vi "log table searching.vi"() -> ()   [LabVIEW 2019, in "database.lvlib"]
uses:
  database.lvlib
panel:
  out "Name":string="Search in Database"
  in  "add 5":bool=TRUE
  in  "add 4":bool=TRUE
  in  "add 3":bool=TRUE
  in  "add 2":bool=TRUE
  in  "add 1":bool=TRUE
  in  "sub 5":bool=TRUE
  in  "sub 4":bool=TRUE
  in  "sub 3":bool=TRUE
  in  "sub 2":bool=TRUE
  in  "sub 1":bool=TRUE
  out "Value String 12":string="Value"
  out "Value String 11":string="Value"
  out "Value String 10":string="Value"
  out "Value String 9":string="Value"
  out "Value String 8":string="Value"
  out "Value String 7":string="Value"
  out "Value String 6":string="Value"
  out "Value String 5":string="Value"
  out "Value String 4":string="Value"
  out "Value String 3":string="Value"
  out "Value String 2":string="Value"
  out "Value String 1":string="Value"
  out "String 4":string="Parameter"
  out "String 3":string="Operation"
  out "String 2":string="Value 2"
  out "String 1":string="Value 1"
  in  "Parameter 1":u16(ring) items=["Choose parameter", "Date", "Time", "Catalog ID"]
  in  "Catalog ID 2":u16
  in  "Catalog ID 1":u64
  in  "Time 1":timestamp format="%<%H:%M:%S>T"
  in  "Time 2":timestamp format="%<%H:%M:%S>T"
  in  "Date 1":timestamp format="%<%Y/%m/%d>T"
  in  "Date 2":timestamp format="%<%Y/%m/%d>T"
  in  "Operator 1":u16(ring) items=["All", "P=V1", "P#V1", "P<V1", "P<=V1", "P>V1", "P>=V1", "V1<P<V2", "V1<=P<V2", "V1<P<=V2", "V1<=P<=V2"]
  in  "Parameter 3":u16(ring) items=["Choose parameter", "Date", "Time", "Catalog ID"]
  in  "Parameter 5":u16(ring) items=["Choose parameter", "Date", "Time", "Catalog ID"]
  in  "Parameter 7":u16(ring) items=["Choose parameter", "Date", "Time", "Catalog ID"]
  in  "Parameter 9":u16(ring) items=["Choose parameter", "Date", "Time", "Catalog ID"]
  in  "Parameter 11":u16(ring) items=["Choose parameter", "Date", "Time", "Catalog ID"]
  in  "Operator 3":u16(ring) items=["All", "P=V1", "P#V1", "P<V1", "P<=V1", "P>V1", "P>=V1", "V1<P<V2", "V1<=P<V2", "V1<P<=V2", "V1<=P<=V2"]
  in  "Catalog ID 3":u64
  in  "Catalog ID 4":u16
  in  "Time 3":timestamp format="%<%H:%M:%S>T"
  in  "Time 4":timestamp format="%<%H:%M:%S>T"
  in  "Date 3":timestamp format="%<%Y/%m/%d>T"
  in  "Date 4":timestamp format="%<%Y/%m/%d>T"
  in  "Catalog ID 5":u64
  in  "Catalog ID 6":u16
  in  "Time 5":timestamp format="%<%H:%M:%S>T"
  in  "Time 6":timestamp format="%<%H:%M:%S>T"
  in  "Date 5":timestamp format="%<%Y/%m/%d>T"
  in  "Date 6":timestamp format="%<%Y/%m/%d>T"
  in  "Operator 5":u16(ring) items=["All", "P=V1", "P#V1", "P<V1", "P<=V1", "P>V1", "P>=V1", "V1<P<V2", "V1<=P<V2", "V1<P<=V2", "V1<=P<=V2"]
  in  "Operator 7":u16(ring) items=["All", "P=V1", "P#V1", "P<V1", "P<=V1", "P>V1", "P>=V1", "V1<P<V2", "V1<=P<V2", "V1<P<=V2", "V1<=P<=V2"]
  in  "Catalog ID 7":u64
  in  "Catalog ID 8":u16
  in  "Time 7":timestamp format="%<%H:%M:%S>T"
  in  "Time 8":timestamp format="%<%H:%M:%S>T"
  in  "Date 7":timestamp format="%<%Y/%m/%d>T"
  in  "Date 8":timestamp format="%<%Y/%m/%d>T"
  in  "Catalog ID 9":u64
  in  "Catalog ID 10":u16
  in  "Time 9":timestamp format="%<%H:%M:%S>T"
  in  "Time 10":timestamp format="%<%H:%M:%S>T"
  in  "Date 9":timestamp format="%<%Y/%m/%d>T"
  in  "Date 10":timestamp format="%<%Y/%m/%d>T"
  in  "Catalog ID 11":u64
  in  "Catalog ID 12":u16
  in  "Time 11":timestamp format="%<%H:%M:%S>T"
  in  "Time 12":timestamp format="%<%H:%M:%S>T"
  in  "Date 11":timestamp format="%<%Y/%m/%d>T"
  in  "Date 12":timestamp format="%<%Y/%m/%d>T"
  in  "Operator 11":u16(ring) items=["All", "P=V1", "P#V1", "P<V1", "P<=V1", "P>V1", "P>=V1", "V1<P<V2", "V1<=P<V2", "V1<P<=V2", "V1<=P<=V2"]
  in  "Operator 9":u16(ring) items=["All", "P=V1", "P#V1", "P<V1", "P<=V1", "P>V1", "P>=V1", "V1<P<V2", "V1<=P<V2", "V1<P<=V2", "V1<=P<=V2"]
  in  "Operator 13":u16(ring) items=["AND", "OR"]
  in  "Operator 14":u16(ring) items=["AND", "OR"]
  in  "Operator 15":u16(ring) items=["AND", "OR"]
  in  "Operator 16":u16(ring) items=["AND", "OR"]
  in  "Operator 17":u16(ring) items=["AND", "OR"]
  out "Query String":string
  in  "OK":bool
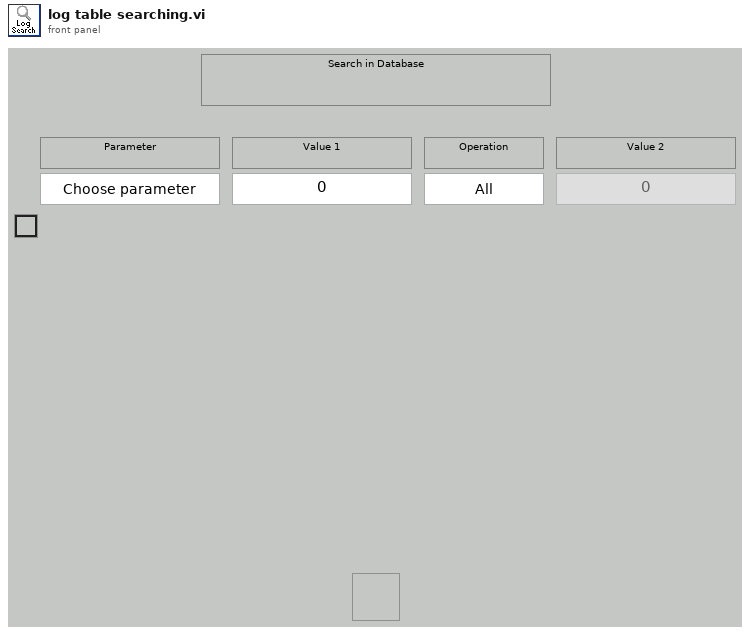
[diagram p1: front panel]
types:
  T1 = enum8{"Enabled", "Disabled", "Disabled and Grayed Out"}
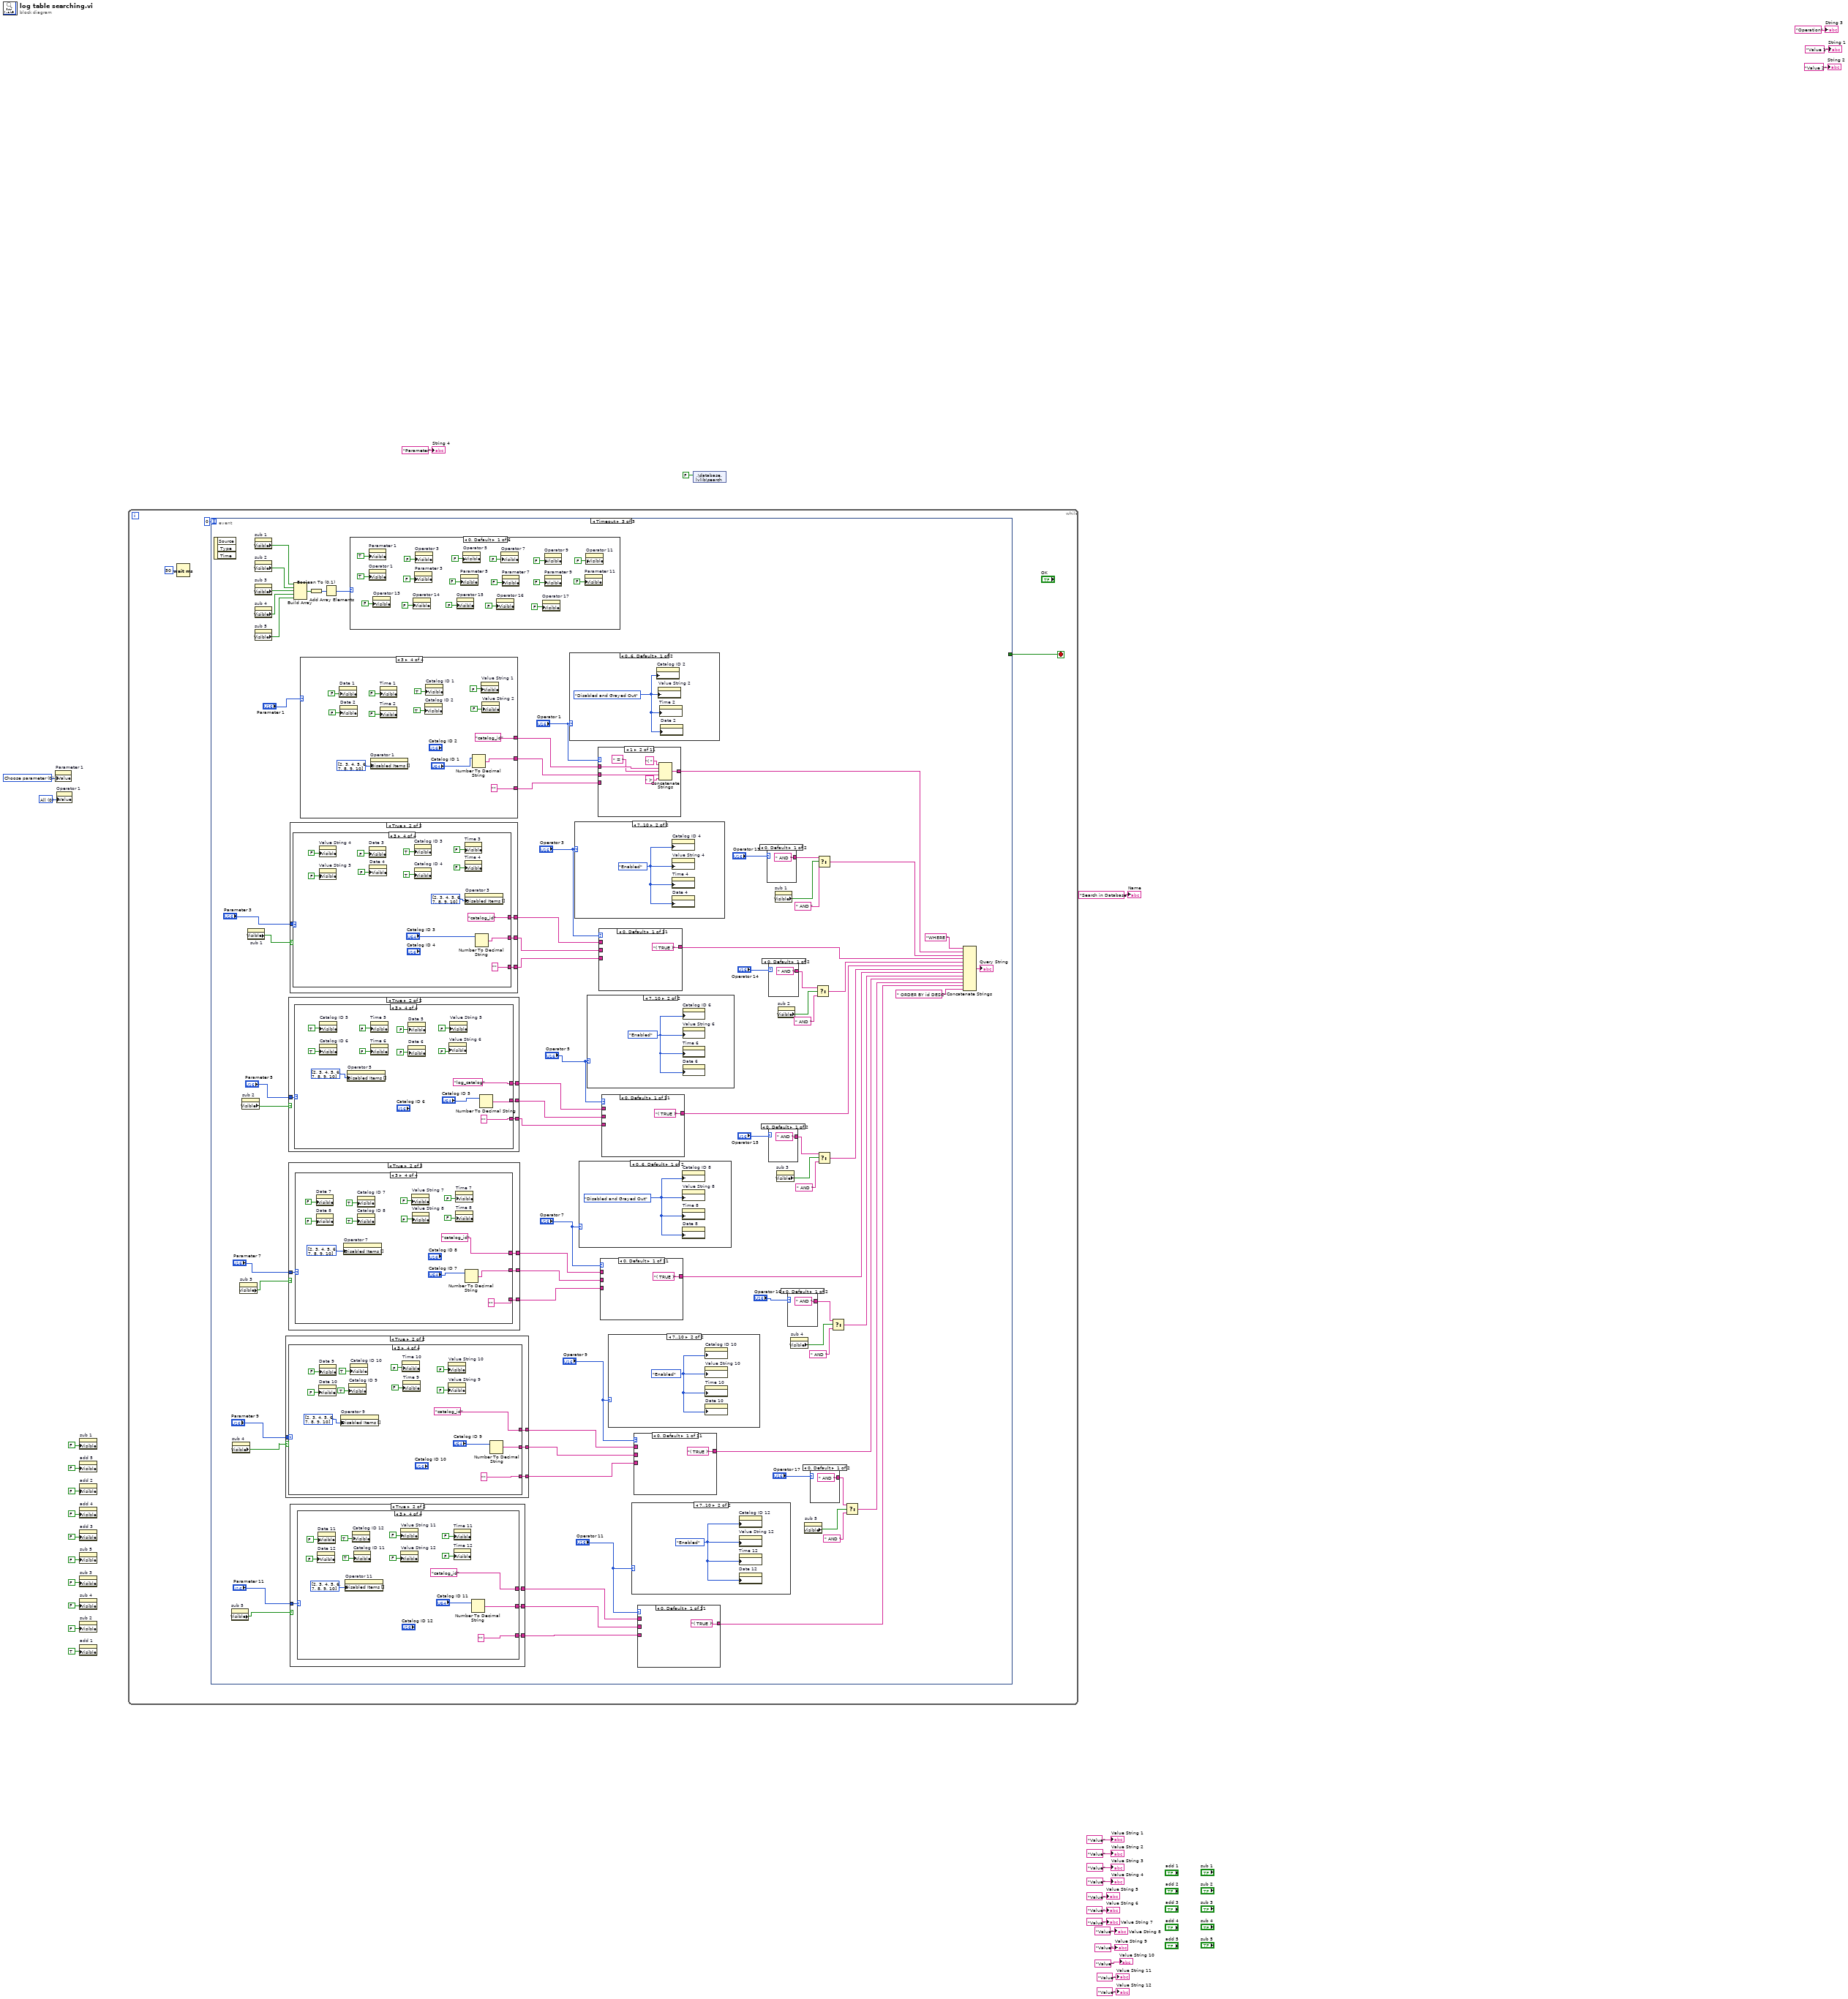
[diagram p0: block diagram]
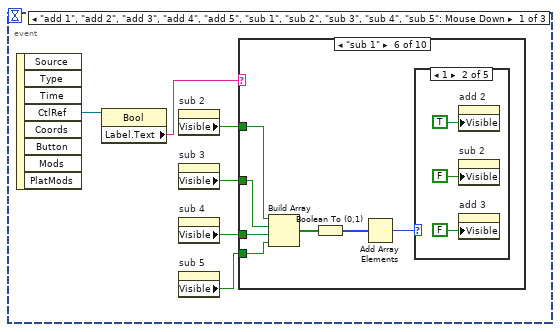
[diagram p2: hidden frame]
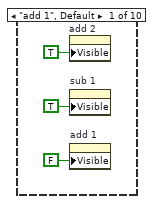
[diagram p3: hidden frame]
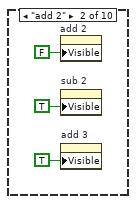
[diagram p4: hidden frame]
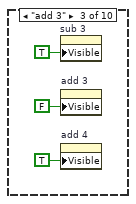
[diagram p5: hidden frame]
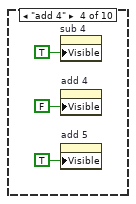
[diagram p6: hidden frame]
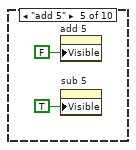
[diagram p7: hidden frame]
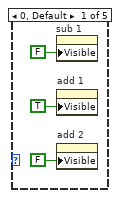
[diagram p8: hidden frame]
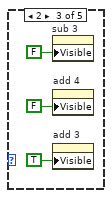
[diagram p9: hidden frame]
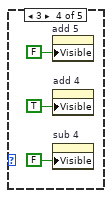
[diagram p10: hidden frame]
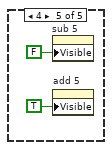
[diagram p11: hidden frame]
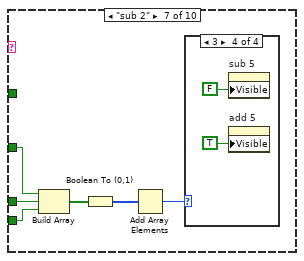
[diagram p12: hidden frame]
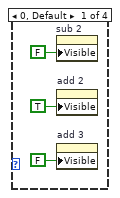
[diagram p13: hidden frame]
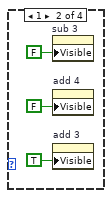
[diagram p14: hidden frame]
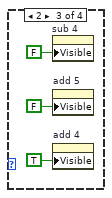
[diagram p15: hidden frame]
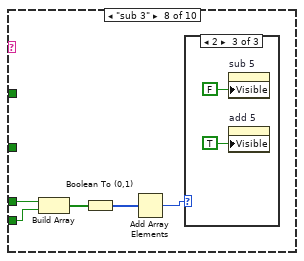
[diagram p16: hidden frame]
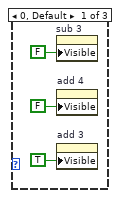
[diagram p17: hidden frame]
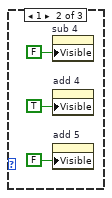
[diagram p18: hidden frame]
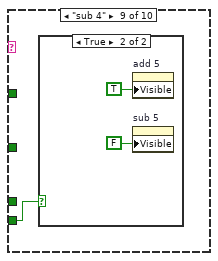
[diagram p19: hidden frame]
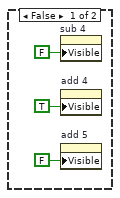
[diagram p20: hidden frame]
diagram:
  w3 = u16 0 items=["All", "P=V1", "P#V1", "P<V1", "P<=V1", "P>V1", "P>=V1", "V1<P<V2", "V1<=P<V2", "V1<P<=V2", "V1<=P<=V2"] ("Operator 1")
  w4 = u16 0 items=["Choose parameter", "Date", "Time", "Disc Situation", "Control Mode", "Camera Situation", "Projector Situation"] ("Parameter 1")
  n1 = property on="Parameter 1" class="Ring (strict)"("Value"=w4) -> ()  [unwired: 2 in, 2 out]
  n2 = property on="Operator 1" class="Ring (strict)"("Value"=w3) -> ()  [unwired: 2 in, 2 out]
  n3 = property on="sub 1" class="Bool"("Visible"=FALSE) -> ()  [unwired: 2 in, 2 out]
  n4 = property on="add 5" class="Bool"("Visible"=FALSE) -> ()  [unwired: 2 in, 2 out]
  n5 = property on="add 2" class="Bool"("Visible"=FALSE) -> ()  [unwired: 2 in, 2 out]
  n6 = property on="add 4" class="Bool"("Visible"=FALSE) -> ()  [unwired: 2 in, 2 out]
  n7 = property on="add 3" class="Bool"("Visible"=FALSE) -> ()  [unwired: 2 in, 2 out]
  n8 = property on="sub 5" class="Bool"("Visible"=FALSE) -> ()  [unwired: 2 in, 2 out]
  n9 = property on="sub 3" class="Bool"("Visible"=FALSE) -> ()  [unwired: 2 in, 2 out]
  n10 = property on="sub 4" class="Bool"("Visible"=FALSE) -> ()  [unwired: 2 in, 2 out]
  n11 = property on="sub 2" class="Bool"("Visible"=FALSE) -> ()  [unwired: 2 in, 2 out]
  n12 = property on="add 1" class="Bool"("Visible"=TRUE) -> ()  [unwired: 2 in, 2 out]
  n13 = while {
    stop <- w31 stop-if-true
    n14 = Wait (ms)(milliseconds to wait=u32 50) -> ()  [unwired: 1 out]
    n15 = event shown="[2] Timeout" {
      selector: _ -> [_ _ _]
      dyn-events: _ -> [_ _ _]
      timeout: 0 -> [_ _ _]
      tunnel: [_ TRUE _] -> w31
      event "add 1", "add 2", "add 3", "add 4", "add 5", "sub 1", "sub 2", "sub 3", "sub 4", "sub 5": Mouse Down {
        n16 = event-data() -> ("CtlRef"=w39:refnum<vi>)  [unwired: 1 in, 7 out]
        n17 = property class="Bool"(reference=w39) -> ("Label.Text"=w38:string)  [unwired: 1 in, 2 out]
        n18 = property on="sub 2" class="Bool"() -> ("Visible"=w37:bool)  [unwired: 2 in, 2 out]
        n19 = property on="sub 3" class="Bool"() -> ("Visible"=w36:bool)  [unwired: 2 in, 2 out]
        n20 = property on="sub 4" class="Bool"() -> ("Visible"=w35:bool)  [unwired: 2 in, 2 out]
        n21 = property on="sub 5" class="Bool"() -> ("Visible"=w34:bool)  [unwired: 2 in, 2 out]
        n22 = case shown="\"sub 1\"" w38 {
          tunnel: w37 -> [_ _ _ _ _ w58 _ _ _ _]
          tunnel: w36 -> [_ _ _ _ _ w57 w78 _ _ _]
          tunnel: w35 -> [_ _ _ _ _ w56 w77 w94 _ _]
          tunnel: w34 -> [_ _ _ _ _ w55 w76 w93 w105 _]
          frame "add 1", Default {
            n23 = property on="add 2" class="Bool"("Visible"=TRUE) -> ()  [unwired: 2 in, 2 out]
            n24 = property on="sub 1" class="Bool"("Visible"=TRUE) -> ()  [unwired: 2 in, 2 out]
            n25 = property on="add 1" class="Bool"("Visible"=FALSE) -> ()  [unwired: 2 in, 2 out]
          }
          frame "add 2" {
            n26 = property on="add 2" class="Bool"("Visible"=FALSE) -> ()  [unwired: 2 in, 2 out]
            n27 = property on="sub 2" class="Bool"("Visible"=TRUE) -> ()  [unwired: 2 in, 2 out]
            n28 = property on="add 3" class="Bool"("Visible"=TRUE) -> ()  [unwired: 2 in, 2 out]
          }
          frame "add 3" {
            n29 = property on="sub 3" class="Bool"("Visible"=TRUE) -> ()  [unwired: 2 in, 2 out]
            n30 = property on="add 3" class="Bool"("Visible"=FALSE) -> ()  [unwired: 2 in, 2 out]
            n31 = property on="add 4" class="Bool"("Visible"=TRUE) -> ()  [unwired: 2 in, 2 out]
          }
          frame "add 4" {
            n32 = property on="sub 4" class="Bool"("Visible"=TRUE) -> ()  [unwired: 2 in, 2 out]
            n33 = property on="add 4" class="Bool"("Visible"=FALSE) -> ()  [unwired: 2 in, 2 out]
            n34 = property on="add 5" class="Bool"("Visible"=TRUE) -> ()  [unwired: 2 in, 2 out]
          }
          frame "add 5" {
            n35 = property on="add 5" class="Bool"("Visible"=FALSE) -> ()  [unwired: 2 in, 2 out]
            n36 = property on="sub 5" class="Bool"("Visible"=TRUE) -> ()  [unwired: 2 in, 2 out]
          }
          frame "sub 1" {
            n37 = Build Array(w58, w57, w56, w55) -> (w54:bool[])
            n38 = Boolean To (0,1)(Boolean=w54) -> (0, 1=w59:i16[])
            n39 = Add Array Elements(numeric array=w59) -> (sum=w60:i16)
            n40 = case shown="1" w60 {
              frame 0, Default {
                n41 = property on="sub 1" class="Bool"("Visible"=FALSE) -> ()  [unwired: 2 in, 2 out]
                n42 = property on="add 1" class="Bool"("Visible"=TRUE) -> ()  [unwired: 2 in, 2 out]
                n43 = property on="add 2" class="Bool"("Visible"=FALSE) -> ()  [unwired: 2 in, 2 out]
              }
              frame 1 {
                n44 = property on="add 2" class="Bool"("Visible"=TRUE) -> ()  [unwired: 2 in, 2 out]
                n45 = property on="sub 2" class="Bool"("Visible"=FALSE) -> ()  [unwired: 2 in, 2 out]
                n46 = property on="add 3" class="Bool"("Visible"=FALSE) -> ()  [unwired: 2 in, 2 out]
              }
              frame 2 {
                n47 = property on="sub 3" class="Bool"("Visible"=FALSE) -> ()  [unwired: 2 in, 2 out]
                n48 = property on="add 4" class="Bool"("Visible"=FALSE) -> ()  [unwired: 2 in, 2 out]
                n49 = property on="add 3" class="Bool"("Visible"=TRUE) -> ()  [unwired: 2 in, 2 out]
              }
              frame 3 {
                n50 = property on="add 5" class="Bool"("Visible"=FALSE) -> ()  [unwired: 2 in, 2 out]
                n51 = property on="add 4" class="Bool"("Visible"=TRUE) -> ()  [unwired: 2 in, 2 out]
                n52 = property on="sub 4" class="Bool"("Visible"=FALSE) -> ()  [unwired: 2 in, 2 out]
              }
              frame 4 {
                n53 = property on="sub 5" class="Bool"("Visible"=FALSE) -> ()  [unwired: 2 in, 2 out]
                n54 = property on="add 5" class="Bool"("Visible"=TRUE) -> ()  [unwired: 2 in, 2 out]
              }
            }
          }
          frame "sub 2" {
            n55 = Build Array(w78, w77, w76) -> (w79:bool[])
            n56 = Boolean To (0,1)(Boolean=w79) -> (0, 1=w80:i16[])
            n57 = Add Array Elements(numeric array=w80) -> (sum=w75:i16)
            n58 = case shown="3" w75 {
              frame 0, Default {
                n59 = property on="sub 2" class="Bool"("Visible"=FALSE) -> ()  [unwired: 2 in, 2 out]
                n60 = property on="add 2" class="Bool"("Visible"=TRUE) -> ()  [unwired: 2 in, 2 out]
                n61 = property on="add 3" class="Bool"("Visible"=FALSE) -> ()  [unwired: 2 in, 2 out]
              }
              frame 1 {
                n62 = property on="sub 3" class="Bool"("Visible"=FALSE) -> ()  [unwired: 2 in, 2 out]
                n63 = property on="add 4" class="Bool"("Visible"=FALSE) -> ()  [unwired: 2 in, 2 out]
                n64 = property on="add 3" class="Bool"("Visible"=TRUE) -> ()  [unwired: 2 in, 2 out]
              }
              frame 2 {
                n65 = property on="sub 4" class="Bool"("Visible"=FALSE) -> ()  [unwired: 2 in, 2 out]
                n66 = property on="add 5" class="Bool"("Visible"=FALSE) -> ()  [unwired: 2 in, 2 out]
                n67 = property on="add 4" class="Bool"("Visible"=TRUE) -> ()  [unwired: 2 in, 2 out]
              }
              frame 3 {
                n68 = property on="sub 5" class="Bool"("Visible"=FALSE) -> ()  [unwired: 2 in, 2 out]
                n69 = property on="add 5" class="Bool"("Visible"=TRUE) -> ()  [unwired: 2 in, 2 out]
              }
            }
          }
          frame "sub 3" {
            n70 = Build Array(w94, w93) -> (w95:bool[])
            n71 = Boolean To (0,1)(Boolean=w95) -> (0, 1=w96:i16[])
            n72 = Add Array Elements(numeric array=w96) -> (sum=w92:i16)
            n73 = case shown="2" w92 {
              frame 0, Default {
                n74 = property on="sub 3" class="Bool"("Visible"=FALSE) -> ()  [unwired: 2 in, 2 out]
                n75 = property on="add 4" class="Bool"("Visible"=FALSE) -> ()  [unwired: 2 in, 2 out]
                n76 = property on="add 3" class="Bool"("Visible"=TRUE) -> ()  [unwired: 2 in, 2 out]
              }
              frame 1 {
                n77 = property on="sub 4" class="Bool"("Visible"=FALSE) -> ()  [unwired: 2 in, 2 out]
                n78 = property on="add 4" class="Bool"("Visible"=TRUE) -> ()  [unwired: 2 in, 2 out]
                n79 = property on="add 5" class="Bool"("Visible"=FALSE) -> ()  [unwired: 2 in, 2 out]
              }
              frame 2 {
                n80 = property on="sub 5" class="Bool"("Visible"=FALSE) -> ()  [unwired: 2 in, 2 out]
                n81 = property on="add 5" class="Bool"("Visible"=TRUE) -> ()  [unwired: 2 in, 2 out]
              }
            }
          }
          frame "sub 4" {
            n82 = case shown="True" w105 {
              frame False {
                n83 = property on="sub 4" class="Bool"("Visible"=FALSE) -> ()  [unwired: 2 in, 2 out]
                n84 = property on="add 4" class="Bool"("Visible"=TRUE) -> ()  [unwired: 2 in, 2 out]
                n85 = property on="add 5" class="Bool"("Visible"=FALSE) -> ()  [unwired: 2 in, 2 out]
              }
              frame True {
                n86 = property on="add 5" class="Bool"("Visible"=TRUE) -> ()  [unwired: 2 in, 2 out]
                n87 = property on="sub 5" class="Bool"("Visible"=FALSE) -> ()  [unwired: 2 in, 2 out]
              }
            }
          }
          frame "sub 5" {
            n88 = property on="sub 5" class="Bool"("Visible"=FALSE) -> ()  [unwired: 2 in, 2 out]
            n89 = property on="add 5" class="Bool"("Visible"=TRUE) -> ()  [unwired: 2 in, 2 out]
          }
        }
      }
      event "OK": Mouse Down {
        n90 = event-data() -> ()  [unwired: 1 in, 8 out]
        n91 = property on="Query String" class="Str"() -> ("Value"=w115:string)  [unwired: 2 in, 2 out]
        n92 = shared-variable ".\\database.lvlib\\Query String"(w115) -> ()  [unwired: 1 in, 1 out]
        n93 = shared-variable ".\\database.lvlib\\search"(TRUE ("search")) -> ()  [unwired: 1 in, 1 out]
      }
      event Timeout {
        n94 = event-data() -> ()  [unwired: 1 in, 3 out]
        n95 = property on="sub 5" class="Bool"() -> ("Visible"=w158:bool)  [unwired: 2 in, 2 out]
        n96 = property on="sub 4" class="Bool"() -> ("Visible"=w159:bool)  [unwired: 2 in, 2 out]
        n97 = property on="sub 3" class="Bool"() -> ("Visible"=w164:bool)  [unwired: 2 in, 2 out]
        n98 = property on="sub 2" class="Bool"() -> ("Visible"=w173:bool)  [unwired: 2 in, 2 out]
        n99 = property on="sub 1" class="Bool"() -> ("Visible"=w174:bool)  [unwired: 2 in, 2 out]
        n100 = property on="sub 1" class="Bool"() -> ("Visible"=w188:bool)  [unwired: 2 in, 2 out]
        n101 = property on="sub 2" class="Bool"() -> ("Visible"=w189:bool)  [unwired: 2 in, 2 out]
        n102 = property on="sub 3" class="Bool"() -> ("Visible"=w190:bool)  [unwired: 2 in, 2 out]
        n103 = property on="sub 4" class="Bool"() -> ("Visible"=w191:bool)  [unwired: 2 in, 2 out]
        n104 = property on="sub 5" class="Bool"() -> ("Visible"=w192:bool)  [unwired: 2 in, 2 out]
        n105 = case shown="True" w159 {
          tunnel: "Parameter 9" -> [_ w456]
          tunnel: ["" ("format string") w455] -> w152
          tunnel: ["" w454] -> w151
          tunnel: ["" ("date/time string") w453] -> w150
          frame False {
            w440 = u16 0 items=["Choose parameter", "Date", "Time", "Catalog ID"] ("Parameter 9")
            w444 = u16 0 items=["All", "P=V1", "P#V1", "P<V1", "P<=V1", "P>V1", "P>=V1", "V1<P<V2", "V1<=P<V2", "V1<P<=V2", "V1<=P<=V2"] ("Operator 9")
            n106 = property on="Date 10" class="AbsTime (strict)"("Visible"=FALSE) -> ()  [unwired: 2 in, 2 out]
            n107 = property on="Date 9" class="AbsTime (strict)"("Visible"=FALSE) -> ()  [unwired: 2 in, 2 out]
            n108 = property on="Catalog ID 9" class="DigNum (strict)"("Visible"=FALSE) -> ()  [unwired: 2 in, 2 out]
            n109 = property on="Catalog ID 10" class="DigNum (strict)"("Visible"=FALSE) -> ()  [unwired: 2 in, 2 out]
            n110 = property on="Parameter 9" class="Ring (strict)"("Value"=w440) -> ()  [unwired: 2 in, 2 out]
            n111 = property on="Operator 9" class="Ring (strict)"("Value"=w444) -> ()  [unwired: 2 in, 2 out]
            n112 = property on="Time 10" class="AbsTime (strict)"("Visible"=FALSE) -> ()  [unwired: 2 in, 2 out]
            n113 = property on="Time 9" class="AbsTime (strict)"("Visible"=FALSE) -> ()  [unwired: 2 in, 2 out]
            n114 = property on="Value String 10" class="Str"("Visible"=FALSE) -> ()  [unwired: 2 in, 2 out]
            n115 = property on="Value String 9" class="Str"("Visible"=FALSE) -> ()  [unwired: 2 in, 2 out]
          }
          frame True {
            n116 = case shown="3" w456 {
              tunnel: ["" ("format string") "date" ("format string") "time" ("format string") "catalog_id" ("format string")] -> w455
              tunnel: ["" w474 w495 w515] -> w454
              tunnel: ["" ("date/time string") w473 w494 "" ("date/time string")] -> w453
              frame 0, Default {
                w457 = u16 0 items=["All", "P=V1", "P#V1", "P<V1", "P<=V1", "P>V1", "P>=V1", "V1<P<V2", "V1<=P<V2", "V1<P<=V2", "V1<=P<=V2"] ("Operator 9")
                n117 = property on="Date 10" class="AbsTime (strict)"("Visible"=FALSE) -> ()  [unwired: 2 in, 2 out]
                n118 = property on="Date 9" class="AbsTime (strict)"("Visible"=FALSE) -> ()  [unwired: 2 in, 2 out]
                n119 = property on="Catalog ID 9" class="DigNum (strict)"("Visible"=FALSE) -> ()  [unwired: 2 in, 2 out]
                n120 = property on="Catalog ID 10" class="DigNum (strict)"("Visible"=FALSE) -> ()  [unwired: 2 in, 2 out]
                n121 = property on="Operator 9" class="Ring (strict)"("Disabled Items []"=i32[] [1, 2, 3, 4, 5, 6, 7, 8, 9, 10], "Value"=w457) -> ()  [unwired: 2 in, 2 out]
                n122 = property on="Time 10" class="AbsTime (strict)"("Visible"=FALSE) -> ()  [unwired: 2 in, 2 out]
                n123 = property on="Time 9" class="AbsTime (strict)"("Visible"=FALSE) -> ()  [unwired: 2 in, 2 out]
                n124 = property on="Value String 10" class="Str"("Visible"=TRUE) -> ()  [unwired: 2 in, 2 out]
                n125 = property on="Value String 9" class="Str"("Visible"=TRUE) -> ()  [unwired: 2 in, 2 out]
              }
              frame 1 {
                n126 = property on="Date 10" class="AbsTime (strict)"("Visible"=TRUE) -> ()  [unwired: 2 in, 2 out]
                n127 = property on="Date 9" class="AbsTime (strict)"("Visible"=TRUE) -> ()  [unwired: 2 in, 2 out]
                n128 = property on="Operator 9" class="Ring (strict)"("Disabled Items []"=i32[] []) -> ()  [unwired: 2 in, 2 out]
                n129 = property on="Catalog ID 9" class="DigNum (strict)"("Visible"=FALSE) -> ()  [unwired: 2 in, 2 out]
                n130 = property on="Catalog ID 10" class="DigNum (strict)"("Visible"=FALSE) -> ()  [unwired: 2 in, 2 out]
                n131 = property on="Time 10" class="AbsTime (strict)"("Visible"=FALSE) -> ()  [unwired: 2 in, 2 out]
                n132 = property on="Time 9" class="AbsTime (strict)"("Visible"=FALSE) -> ()  [unwired: 2 in, 2 out]
                n133 = Format Date/Time String(time format string (%c)="%Y/%m/%d", seconds (now)="Date 9") -> (date/time string=w482:string)  [unwired: 1 in]
                n134 = Format Date/Time String(time format string (%c)="%Y/%m/%d", seconds (now)="Date 10") -> (date/time string=w481:string)  [unwired: 1 in]
                n135 = property on="Value String 10" class="Str"("Visible"=FALSE) -> ()  [unwired: 2 in, 2 out]
                n136 = property on="Value String 9" class="Str"("Visible"=FALSE) -> ()  [unwired: 2 in, 2 out]
                n137 = Concatenate Strings("'" ("string"), w482, "'" ("string")) -> (w474:string)
                n138 = Concatenate Strings("'" ("string"), w481, "'" ("string")) -> (w473:string)
              }
              frame 2 {
                n139 = property on="Date 10" class="AbsTime (strict)"("Visible"=FALSE) -> ()  [unwired: 2 in, 2 out]
                n140 = property on="Date 9" class="AbsTime (strict)"("Visible"=FALSE) -> ()  [unwired: 2 in, 2 out]
                n141 = property on="Operator 9" class="Ring (strict)"("Disabled Items []"=i32[] []) -> ()  [unwired: 2 in, 2 out]
                n142 = property on="Catalog ID 9" class="DigNum (strict)"("Visible"=FALSE) -> ()  [unwired: 2 in, 2 out]
                n143 = property on="Catalog ID 10" class="DigNum (strict)"("Visible"=FALSE) -> ()  [unwired: 2 in, 2 out]
                n144 = property on="Time 10" class="AbsTime (strict)"("Visible"=TRUE) -> ()  [unwired: 2 in, 2 out]
                n145 = property on="Time 9" class="AbsTime (strict)"("Visible"=TRUE) -> ()  [unwired: 2 in, 2 out]
                n146 = property on="Value String 10" class="Str"("Visible"=FALSE) -> ()  [unwired: 2 in, 2 out]
                n147 = property on="Value String 9" class="Str"("Visible"=FALSE) -> ()  [unwired: 2 in, 2 out]
                n148 = Format Date/Time String(time format string (%c)="%H:%M:%S", seconds (now)="Time 9") -> (date/time string=w504:string)  [unwired: 1 in]
                n149 = Format Date/Time String(time format string (%c)="%H:%M:%S", seconds (now)="Time 10") -> (date/time string=w503:string)  [unwired: 1 in]
                n150 = Concatenate Strings("'" ("string"), w504, "'" ("string")) -> (w495:string)
                n151 = Concatenate Strings("'" ("string"), w503, "'" ("string")) -> (w494:string)
              }
              frame 3 {
                n152 = property on="Date 10" class="AbsTime (strict)"("Visible"=FALSE) -> ()  [unwired: 2 in, 2 out]
                n153 = property on="Date 9" class="AbsTime (strict)"("Visible"=FALSE) -> ()  [unwired: 2 in, 2 out]
                n154 = property on="Operator 9" class="Ring (strict)"("Disabled Items []"=i32[] [2, 3, 4, 5, 6, 7, 8, 9, 10]) -> ()  [unwired: 2 in, 2 out]
                n155 = property on="Catalog ID 9" class="DigNum (strict)"("Visible"=TRUE) -> ()  [unwired: 2 in, 2 out]
                n156 = property on="Catalog ID 10" class="DigNum (strict)"("Visible"=TRUE) -> ()  [unwired: 2 in, 2 out]
                n157 = property on="Time 10" class="AbsTime (strict)"("Visible"=FALSE) -> ()  [unwired: 2 in, 2 out]
                n158 = property on="Time 9" class="AbsTime (strict)"("Visible"=FALSE) -> ()  [unwired: 2 in, 2 out]
                n159 = property on="Value String 10" class="Str"("Visible"=FALSE) -> ()  [unwired: 2 in, 2 out]
                n160 = property on="Value String 9" class="Str"("Visible"=FALSE) -> ()  [unwired: 2 in, 2 out]
                n161 = Number To Decimal String(number="Catalog ID 9") -> (decimal integer string=w515:string)  [unwired: 1 in]
              }
            }
          }
        }
        n162 = case shown="True" w173 {
          tunnel: "Parameter 5" -> [_ w853]
          tunnel: ["" ("format string") w852] -> w167
          tunnel: ["" ("date/time string") w851] -> w166
          tunnel: ["" ("date/time string") w850] -> w165
          frame False {
            w837 = u16 0 items=["Choose parameter", "Date", "Time", "Catalog ID"] ("Parameter 5")
            w841 = u16 0 items=["All", "P=V1", "P#V1", "P<V1", "P<=V1", "P>V1", "P>=V1", "V1<P<V2", "V1<=P<V2", "V1<P<=V2", "V1<=P<=V2"] ("Operator 5")
            n163 = property on="Catalog ID 5" class="DigNum (strict)"("Visible"=FALSE) -> ()  [unwired: 2 in, 2 out]
            n164 = property on="Catalog ID 6" class="DigNum (strict)"("Visible"=FALSE) -> ()  [unwired: 2 in, 2 out]
            n165 = property on="Time 5" class="AbsTime (strict)"("Visible"=FALSE) -> ()  [unwired: 2 in, 2 out]
            n166 = property on="Time 6" class="AbsTime (strict)"("Visible"=FALSE) -> ()  [unwired: 2 in, 2 out]
            n167 = property on="Date 5" class="AbsTime (strict)"("Visible"=FALSE) -> ()  [unwired: 2 in, 2 out]
            n168 = property on="Date 6" class="AbsTime (strict)"("Visible"=FALSE) -> ()  [unwired: 2 in, 2 out]
            n169 = property on="Operator 5" class="Ring (strict)"("Value"=w841) -> ()  [unwired: 2 in, 2 out]
            n170 = property on="Parameter 5" class="Ring (strict)"("Value"=w837) -> ()  [unwired: 2 in, 2 out]
            n171 = property on="Value String 6" class="Str"("Visible"=FALSE) -> ()  [unwired: 2 in, 2 out]
            n172 = property on="Value String 5" class="Str"("Visible"=FALSE) -> ()  [unwired: 2 in, 2 out]
          }
          frame True {
            n173 = case shown="3" w853 {
              tunnel: ["" ("format string") "date" ("format string") "time" ("format string") "log_catalog" ("format string")] -> w852
              tunnel: ["" ("date/time string") w868 w892 w912] -> w851
              tunnel: ["" ("date/time string") w867 w891 "" ("date/time string")] -> w850
              frame 0, Default {
                w854 = u16 0 items=["All", "P=V1", "P#V1", "P<V1", "P<=V1", "P>V1", "P>=V1", "V1<P<V2", "V1<=P<V2", "V1<P<=V2", "V1<=P<=V2"] ("Operator 5")
                n174 = property on="Catalog ID 5" class="DigNum (strict)"("Visible"=FALSE) -> ()  [unwired: 2 in, 2 out]
                n175 = property on="Catalog ID 6" class="DigNum (strict)"("Visible"=FALSE) -> ()  [unwired: 2 in, 2 out]
                n176 = property on="Operator 5" class="Ring (strict)"("Disabled Items []"=i32[] [1, 2, 3, 4, 5, 6, 7, 8, 9, 10], "Value"=w854) -> ()  [unwired: 2 in, 2 out]
                n177 = property on="Time 5" class="AbsTime (strict)"("Visible"=FALSE) -> ()  [unwired: 2 in, 2 out]
                n178 = property on="Time 6" class="AbsTime (strict)"("Visible"=FALSE) -> ()  [unwired: 2 in, 2 out]
                n179 = property on="Date 5" class="AbsTime (strict)"("Visible"=FALSE) -> ()  [unwired: 2 in, 2 out]
                n180 = property on="Date 6" class="AbsTime (strict)"("Visible"=FALSE) -> ()  [unwired: 2 in, 2 out]
                n181 = property on="Value String 6" class="Str"("Visible"=TRUE) -> ()  [unwired: 2 in, 2 out]
                n182 = property on="Value String 5" class="Str"("Visible"=TRUE) -> ()  [unwired: 2 in, 2 out]
              }
              frame 1 {
                n183 = property on="Catalog ID 5" class="DigNum (strict)"("Visible"=FALSE) -> ()  [unwired: 2 in, 2 out]
                n184 = property on="Catalog ID 6" class="DigNum (strict)"("Visible"=FALSE) -> ()  [unwired: 2 in, 2 out]
                n185 = property on="Operator 5" class="Ring (strict)"("Disabled Items []"=i32[] []) -> ()  [unwired: 2 in, 2 out]
                n186 = property on="Time 5" class="AbsTime (strict)"("Visible"=FALSE) -> ()  [unwired: 2 in, 2 out]
                n187 = property on="Time 6" class="AbsTime (strict)"("Visible"=FALSE) -> ()  [unwired: 2 in, 2 out]
                n188 = property on="Date 5" class="AbsTime (strict)"("Visible"=TRUE) -> ()  [unwired: 2 in, 2 out]
                n189 = property on="Date 6" class="AbsTime (strict)"("Visible"=TRUE) -> ()  [unwired: 2 in, 2 out]
                n190 = Format Date/Time String(time format string (%c)="%Y/%m/%d", seconds (now)="Date 6") -> (date/time string=w872:string)  [unwired: 1 in]
                n191 = Format Date/Time String(time format string (%c)="%Y/%m/%d", seconds (now)="Date 5") -> (date/time string=w873:string)  [unwired: 1 in]
                n192 = property on="Value String 6" class="Str"("Visible"=FALSE) -> ()  [unwired: 2 in, 2 out]
                n193 = property on="Value String 5" class="Str"("Visible"=FALSE) -> ()  [unwired: 2 in, 2 out]
                n194 = Concatenate Strings("'" ("string"), w873, "'" ("string")) -> (w868:string)
                n195 = Concatenate Strings("'" ("string"), w872, "'" ("string")) -> (w867:string)
              }
              frame 2 {
                n196 = property on="Catalog ID 5" class="DigNum (strict)"("Visible"=FALSE) -> ()  [unwired: 2 in, 2 out]
                n197 = property on="Catalog ID 6" class="DigNum (strict)"("Visible"=FALSE) -> ()  [unwired: 2 in, 2 out]
                n198 = property on="Operator 5" class="Ring (strict)"("Disabled Items []"=i32[] []) -> ()  [unwired: 2 in, 2 out]
                n199 = property on="Time 5" class="AbsTime (strict)"("Visible"=TRUE) -> ()  [unwired: 2 in, 2 out]
                n200 = property on="Time 6" class="AbsTime (strict)"("Visible"=TRUE) -> ()  [unwired: 2 in, 2 out]
                n201 = property on="Date 5" class="AbsTime (strict)"("Visible"=FALSE) -> ()  [unwired: 2 in, 2 out]
                n202 = property on="Date 6" class="AbsTime (strict)"("Visible"=FALSE) -> ()  [unwired: 2 in, 2 out]
                n203 = Format Date/Time String(time format string (%c)="%H:%M:%S", seconds (now)="Time 5") -> (date/time string=w889:string)  [unwired: 1 in]
                n204 = Format Date/Time String(time format string (%c)="%H:%M:%S", seconds (now)="Time 6") -> (date/time string=w890:string)  [unwired: 1 in]
                n205 = property on="Value String 6" class="Str"("Visible"=FALSE) -> ()  [unwired: 2 in, 2 out]
                n206 = property on="Value String 5" class="Str"("Visible"=FALSE) -> ()  [unwired: 2 in, 2 out]
                n207 = Concatenate Strings("'" ("string"), w889, "'" ("string")) -> (w892:string)
                n208 = Concatenate Strings("'" ("string"), w890, "'" ("string")) -> (w891:string)
              }
              frame 3 {
                n209 = property on="Catalog ID 5" class="DigNum (strict)"("Visible"=TRUE) -> ()  [unwired: 2 in, 2 out]
                n210 = property on="Catalog ID 6" class="DigNum (strict)"("Visible"=TRUE) -> ()  [unwired: 2 in, 2 out]
                n211 = property on="Operator 5" class="Ring (strict)"("Disabled Items []"=i32[] [2, 3, 4, 5, 6, 7, 8, 9, 10]) -> ()  [unwired: 2 in, 2 out]
                n212 = property on="Time 5" class="AbsTime (strict)"("Visible"=FALSE) -> ()  [unwired: 2 in, 2 out]
                n213 = property on="Time 6" class="AbsTime (strict)"("Visible"=FALSE) -> ()  [unwired: 2 in, 2 out]
                n214 = property on="Date 5" class="AbsTime (strict)"("Visible"=FALSE) -> ()  [unwired: 2 in, 2 out]
                n215 = property on="Date 6" class="AbsTime (strict)"("Visible"=FALSE) -> ()  [unwired: 2 in, 2 out]
                n216 = property on="Value String 6" class="Str"("Visible"=FALSE) -> ()  [unwired: 2 in, 2 out]
                n217 = property on="Value String 5" class="Str"("Visible"=FALSE) -> ()  [unwired: 2 in, 2 out]
                n218 = Number To Decimal String(number="Catalog ID 5") -> (decimal integer string=w912:string)  [unwired: 1 in]
              }
            }
          }
        }
        n219 = case shown="True" w164 {
          tunnel: "Parameter 7" -> [_ w618]
          tunnel: ["" ("format string") w617] -> w162
          tunnel: ["" w616] -> w161
          tunnel: ["" ("date/time string") w615] -> w160
          frame False {
            w602 = u16 0 items=["Choose parameter", "Date", "Time", "Catalog ID"] ("Parameter 7")
            w606 = u16 0 items=["All", "P=V1", "P#V1", "P<V1", "P<=V1", "P>V1", "P>=V1", "V1<P<V2", "V1<=P<V2", "V1<P<=V2", "V1<=P<=V2"] ("Operator 7")
            n220 = property on="Date 7" class="AbsTime (strict)"("Visible"=FALSE) -> ()  [unwired: 2 in, 2 out]
            n221 = property on="Date 8" class="AbsTime (strict)"("Visible"=FALSE) -> ()  [unwired: 2 in, 2 out]
            n222 = property on="Time 7" class="AbsTime (strict)"("Visible"=FALSE) -> ()  [unwired: 2 in, 2 out]
            n223 = property on="Time 8" class="AbsTime (strict)"("Visible"=FALSE) -> ()  [unwired: 2 in, 2 out]
            n224 = property on="Catalog ID 7" class="DigNum (strict)"("Visible"=FALSE) -> ()  [unwired: 2 in, 2 out]
            n225 = property on="Catalog ID 8" class="DigNum (strict)"("Visible"=FALSE) -> ()  [unwired: 2 in, 2 out]
            n226 = property on="Operator 7" class="Ring (strict)"("Value"=w606) -> ()  [unwired: 2 in, 2 out]
            n227 = property on="Parameter 7" class="Ring (strict)"("Value"=w602) -> ()  [unwired: 2 in, 2 out]
            n228 = property on="Value String 7" class="Str"("Visible"=FALSE) -> ()  [unwired: 2 in, 2 out]
            n229 = property on="Value String 8" class="Str"("Visible"=FALSE) -> ()  [unwired: 2 in, 2 out]
          }
          frame True {
            n230 = case shown="3" w618 {
              tunnel: ["" ("format string") "date" ("format string") "time" ("format string") "catalog_id" ("format string")] -> w617
              tunnel: ["" w635 w655 w676] -> w616
              tunnel: ["" ("date/time string") w634 w654 "" ("date/time string")] -> w615
              frame 0, Default {
                w619 = u16 0 items=["All", "P=V1", "P#V1", "P<V1", "P<=V1", "P>V1", "P>=V1", "V1<P<V2", "V1<=P<V2", "V1<P<=V2", "V1<=P<=V2"] ("Operator 7")
                n231 = property on="Date 7" class="AbsTime (strict)"("Visible"=FALSE) -> ()  [unwired: 2 in, 2 out]
                n232 = property on="Date 8" class="AbsTime (strict)"("Visible"=FALSE) -> ()  [unwired: 2 in, 2 out]
                n233 = property on="Catalog ID 7" class="DigNum (strict)"("Visible"=FALSE) -> ()  [unwired: 2 in, 2 out]
                n234 = property on="Catalog ID 8" class="DigNum (strict)"("Visible"=FALSE) -> ()  [unwired: 2 in, 2 out]
                n235 = property on="Operator 7" class="Ring (strict)"("Disabled Items []"=i32[] [1, 2, 3, 4, 5, 6, 7, 8, 9, 10], "Value"=w619) -> ()  [unwired: 2 in, 2 out]
                n236 = property on="Value String 7" class="Str"("Visible"=TRUE) -> ()  [unwired: 2 in, 2 out]
                n237 = property on="Value String 8" class="Str"("Visible"=TRUE) -> ()  [unwired: 2 in, 2 out]
                n238 = property on="Time 7" class="AbsTime (strict)"("Visible"=FALSE) -> ()  [unwired: 2 in, 2 out]
                n239 = property on="Time 8" class="AbsTime (strict)"("Visible"=FALSE) -> ()  [unwired: 2 in, 2 out]
              }
              frame 1 {
                n240 = property on="Date 7" class="AbsTime (strict)"("Visible"=TRUE) -> ()  [unwired: 2 in, 2 out]
                n241 = property on="Date 8" class="AbsTime (strict)"("Visible"=TRUE) -> ()  [unwired: 2 in, 2 out]
                n242 = property on="Operator 7" class="Ring (strict)"("Disabled Items []"=i32[] []) -> ()  [unwired: 2 in, 2 out]
                n243 = property on="Catalog ID 7" class="DigNum (strict)"("Visible"=FALSE) -> ()  [unwired: 2 in, 2 out]
                n244 = property on="Catalog ID 8" class="DigNum (strict)"("Visible"=FALSE) -> ()  [unwired: 2 in, 2 out]
                n245 = property on="Value String 7" class="Str"("Visible"=FALSE) -> ()  [unwired: 2 in, 2 out]
                n246 = property on="Value String 8" class="Str"("Visible"=FALSE) -> ()  [unwired: 2 in, 2 out]
                n247 = property on="Time 7" class="AbsTime (strict)"("Visible"=FALSE) -> ()  [unwired: 2 in, 2 out]
                n248 = property on="Time 8" class="AbsTime (strict)"("Visible"=FALSE) -> ()  [unwired: 2 in, 2 out]
                n249 = Format Date/Time String(time format string (%c)="%Y/%m/%d", seconds (now)="Date 8") -> (date/time string=w644:string)  [unwired: 1 in]
                n250 = Format Date/Time String(time format string (%c)="%Y/%m/%d", seconds (now)="Date 7") -> (date/time string=w643:string)  [unwired: 1 in]
                n251 = Concatenate Strings("'" ("string"), w643, "'" ("string")) -> (w635:string)
                n252 = Concatenate Strings("'" ("string"), w644, "'" ("string")) -> (w634:string)
              }
              frame 2 {
                n253 = property on="Date 7" class="AbsTime (strict)"("Visible"=FALSE) -> ()  [unwired: 2 in, 2 out]
                n254 = property on="Date 8" class="AbsTime (strict)"("Visible"=FALSE) -> ()  [unwired: 2 in, 2 out]
                n255 = property on="Operator 7" class="Ring (strict)"("Disabled Items []"=i32[] []) -> ()  [unwired: 2 in, 2 out]
                n256 = property on="Catalog ID 7" class="DigNum (strict)"("Visible"=FALSE) -> ()  [unwired: 2 in, 2 out]
                n257 = property on="Catalog ID 8" class="DigNum (strict)"("Visible"=FALSE) -> ()  [unwired: 2 in, 2 out]
                n258 = property on="Value String 7" class="Str"("Visible"=FALSE) -> ()  [unwired: 2 in, 2 out]
                n259 = property on="Value String 8" class="Str"("Visible"=FALSE) -> ()  [unwired: 2 in, 2 out]
                n260 = Format Date/Time String(time format string (%c)="%H:%M:%S", seconds (now)="Time 8") -> (date/time string=w666:string)  [unwired: 1 in]
                n261 = Format Date/Time String(time format string (%c)="%H:%M:%S", seconds (now)="Time 7") -> (date/time string=w665:string)  [unwired: 1 in]
                n262 = property on="Time 7" class="AbsTime (strict)"("Visible"=TRUE) -> ()  [unwired: 2 in, 2 out]
                n263 = property on="Time 8" class="AbsTime (strict)"("Visible"=TRUE) -> ()  [unwired: 2 in, 2 out]
                n264 = Concatenate Strings("'" ("string"), w666, "'" ("string")) -> (w655:string)
                n265 = Concatenate Strings("'" ("string"), w665, "'" ("string")) -> (w654:string)
              }
              frame 3 {
                n266 = property on="Date 7" class="AbsTime (strict)"("Visible"=FALSE) -> ()  [unwired: 2 in, 2 out]
                n267 = property on="Date 8" class="AbsTime (strict)"("Visible"=FALSE) -> ()  [unwired: 2 in, 2 out]
                n268 = property on="Operator 7" class="Ring (strict)"("Disabled Items []"=i32[] [2, 3, 4, 5, 6, 7, 8, 9, 10]) -> ()  [unwired: 2 in, 2 out]
                n269 = property on="Catalog ID 7" class="DigNum (strict)"("Visible"=TRUE) -> ()  [unwired: 2 in, 2 out]
                n270 = property on="Catalog ID 8" class="DigNum (strict)"("Visible"=TRUE) -> ()  [unwired: 2 in, 2 out]
                n271 = property on="Value String 7" class="Str"("Visible"=FALSE) -> ()  [unwired: 2 in, 2 out]
                n272 = property on="Value String 8" class="Str"("Visible"=FALSE) -> ()  [unwired: 2 in, 2 out]
                n273 = property on="Time 7" class="AbsTime (strict)"("Visible"=FALSE) -> ()  [unwired: 2 in, 2 out]
                n274 = property on="Time 8" class="AbsTime (strict)"("Visible"=FALSE) -> ()  [unwired: 2 in, 2 out]
                n275 = Number To Decimal String(number="Catalog ID 7") -> (decimal integer string=w676:string)  [unwired: 1 in]
              }
            }
          }
        }
        n276 = case shown="True" w174 {
          tunnel: "Parameter 3" -> [_ w942]
          tunnel: ["" ("format string") w941] -> w171
          tunnel: ["" ("date/time string") w940] -> w170
          tunnel: ["" ("date/time string") w939] -> w169
          frame False {
            w926 = u16 0 items=["Choose parameter", "Date", "Time", "Catalog ID"] ("Parameter 3")
            w927 = u16 0 items=["All", "P=V1", "P#V1", "P<V1", "P<=V1", "P>V1", "P>=V1", "V1<P<V2", "V1<=P<V2", "V1<P<=V2", "V1<=P<=V2"] ("Operator 3")
            n277 = property on="Value String 4" class="Str"("Visible"=FALSE) -> ()  [unwired: 2 in, 2 out]
            n278 = property on="Value String 3" class="Str"("Visible"=FALSE) -> ()  [unwired: 2 in, 2 out]
            n279 = property on="Date 3" class="AbsTime (strict)"("Visible"=FALSE) -> ()  [unwired: 2 in, 2 out]
            n280 = property on="Date 4" class="AbsTime (strict)"("Visible"=FALSE) -> ()  [unwired: 2 in, 2 out]
            n281 = property on="Parameter 3" class="Ring (strict)"("Value"=w926) -> ()  [unwired: 2 in, 2 out]
            n282 = property on="Catalog ID 3" class="DigNum (strict)"("Visible"=FALSE) -> ()  [unwired: 2 in, 2 out]
            n283 = property on="Catalog ID 4" class="DigNum (strict)"("Visible"=FALSE) -> ()  [unwired: 2 in, 2 out]
            n284 = property on="Operator 3" class="Ring (strict)"("Value"=w927) -> ()  [unwired: 2 in, 2 out]
            n285 = property on="Time 3" class="AbsTime (strict)"("Visible"=FALSE) -> ()  [unwired: 2 in, 2 out]
            n286 = property on="Time 4" class="AbsTime (strict)"("Visible"=FALSE) -> ()  [unwired: 2 in, 2 out]
          }
          frame True {
            n287 = case shown="3" w942 {
              tunnel: ["" ("format string") "date" ("format string") "time" ("format string") "catalog_id" ("format string")] -> w941
              tunnel: ["" ("date/time string") w957 w981 w1000] -> w940
              tunnel: ["" ("date/time string") w956 w980 "" ("date/time string")] -> w939
              frame 0, Default {
                w943 = u16 0 items=["All", "P=V1", "P#V1", "P<V1", "P<=V1", "P>V1", "P>=V1", "V1<P<V2", "V1<=P<V2", "V1<P<=V2", "V1<=P<=V2"] ("Operator 3")
                n288 = property on="Value String 4" class="Str"("Visible"=TRUE) -> ()  [unwired: 2 in, 2 out]
                n289 = property on="Value String 3" class="Str"("Visible"=TRUE) -> ()  [unwired: 2 in, 2 out]
                n290 = property on="Date 3" class="AbsTime (strict)"("Visible"=FALSE) -> ()  [unwired: 2 in, 2 out]
                n291 = property on="Date 4" class="AbsTime (strict)"("Visible"=FALSE) -> ()  [unwired: 2 in, 2 out]
                n292 = property on="Operator 3" class="Ring (strict)"("Disabled Items []"=i32[] [1, 2, 3, 4, 5, 6, 7, 8, 9, 10], "Value"=w943) -> ()  [unwired: 2 in, 2 out]
                n293 = property on="Catalog ID 3" class="DigNum (strict)"("Visible"=FALSE) -> ()  [unwired: 2 in, 2 out]
                n294 = property on="Catalog ID 4" class="DigNum (strict)"("Visible"=FALSE) -> ()  [unwired: 2 in, 2 out]
                n295 = property on="Time 3" class="AbsTime (strict)"("Visible"=FALSE) -> ()  [unwired: 2 in, 2 out]
                n296 = property on="Time 4" class="AbsTime (strict)"("Visible"=FALSE) -> ()  [unwired: 2 in, 2 out]
              }
              frame 1 {
                n297 = property on="Value String 4" class="Str"("Visible"=FALSE) -> ()  [unwired: 2 in, 2 out]
                n298 = property on="Value String 3" class="Str"("Visible"=FALSE) -> ()  [unwired: 2 in, 2 out]
                n299 = property on="Date 3" class="AbsTime (strict)"("Visible"=TRUE) -> ()  [unwired: 2 in, 2 out]
                n300 = property on="Date 4" class="AbsTime (strict)"("Visible"=TRUE) -> ()  [unwired: 2 in, 2 out]
                n301 = Format Date/Time String(time format string (%c)="%Y/%m/%d", seconds (now)="Date 4") -> (date/time string=w968:string)  [unwired: 1 in]
                n302 = Format Date/Time String(time format string (%c)="%Y/%m/%d", seconds (now)="Date 3") -> (date/time string=w967:string)  [unwired: 1 in]
                n303 = property on="Catalog ID 3" class="DigNum (strict)"("Visible"=FALSE) -> ()  [unwired: 2 in, 2 out]
                n304 = property on="Catalog ID 4" class="DigNum (strict)"("Visible"=FALSE) -> ()  [unwired: 2 in, 2 out]
                n305 = Concatenate Strings("'" ("string"), w967, "'" ("string")) -> (w957:string)
                n306 = Concatenate Strings("'" ("string"), w968, "'" ("string")) -> (w956:string)
                n307 = property on="Time 3" class="AbsTime (strict)"("Visible"=FALSE) -> ()  [unwired: 2 in, 2 out]
                n308 = property on="Time 4" class="AbsTime (strict)"("Visible"=FALSE) -> ()  [unwired: 2 in, 2 out]
                n309 = property on="Operator 3" class="Ring (strict)"("Disabled Items []"=i32[] []) -> ()  [unwired: 2 in, 2 out]
              }
              frame 2 {
                n310 = property on="Value String 4" class="Str"("Visible"=FALSE) -> ()  [unwired: 2 in, 2 out]
                n311 = property on="Value String 3" class="Str"("Visible"=FALSE) -> ()  [unwired: 2 in, 2 out]
                n312 = property on="Operator 3" class="Ring (strict)"("Disabled Items []"=i32[] []) -> ()  [unwired: 2 in, 2 out]
                n313 = property on="Date 3" class="AbsTime (strict)"("Visible"=FALSE) -> ()  [unwired: 2 in, 2 out]
                n314 = property on="Date 4" class="AbsTime (strict)"("Visible"=FALSE) -> ()  [unwired: 2 in, 2 out]
                n315 = property on="Catalog ID 3" class="DigNum (strict)"("Visible"=FALSE) -> ()  [unwired: 2 in, 2 out]
                n316 = property on="Catalog ID 4" class="DigNum (strict)"("Visible"=FALSE) -> ()  [unwired: 2 in, 2 out]
                n317 = Format Date/Time String(time format string (%c)="%H:%M:%S", seconds (now)="Time 3") -> (date/time string=w978:string)  [unwired: 1 in]
                n318 = Format Date/Time String(time format string (%c)="%H:%M:%S", seconds (now)="Time 4") -> (date/time string=w979:string)  [unwired: 1 in]
                n319 = property on="Time 3" class="AbsTime (strict)"("Visible"=TRUE) -> ()  [unwired: 2 in, 2 out]
                n320 = property on="Time 4" class="AbsTime (strict)"("Visible"=TRUE) -> ()  [unwired: 2 in, 2 out]
                n321 = Concatenate Strings("'" ("string"), w978, "'" ("string")) -> (w981:string)
                n322 = Concatenate Strings("'" ("string"), w979, "'" ("string")) -> (w980:string)
              }
              frame 3 {
                n323 = property on="Value String 4" class="Str"("Visible"=FALSE) -> ()  [unwired: 2 in, 2 out]
                n324 = property on="Value String 3" class="Str"("Visible"=FALSE) -> ()  [unwired: 2 in, 2 out]
                n325 = property on="Date 3" class="AbsTime (strict)"("Visible"=FALSE) -> ()  [unwired: 2 in, 2 out]
                n326 = property on="Date 4" class="AbsTime (strict)"("Visible"=FALSE) -> ()  [unwired: 2 in, 2 out]
                n327 = property on="Catalog ID 3" class="DigNum (strict)"("Visible"=TRUE) -> ()  [unwired: 2 in, 2 out]
                n328 = property on="Catalog ID 4" class="DigNum (strict)"("Visible"=TRUE) -> ()  [unwired: 2 in, 2 out]
                n329 = property on="Time 3" class="AbsTime (strict)"("Visible"=FALSE) -> ()  [unwired: 2 in, 2 out]
                n330 = property on="Time 4" class="AbsTime (strict)"("Visible"=FALSE) -> ()  [unwired: 2 in, 2 out]
                n331 = property on="Operator 3" class="Ring (strict)"("Disabled Items []"=i32[] [2, 3, 4, 5, 6, 7, 8, 9, 10]) -> ()  [unwired: 2 in, 2 out]
                n332 = Number To Decimal String(number="Catalog ID 3") -> (decimal integer string=w1000:string)  [unwired: 1 in]
              }
            }
          }
        }
        n333 = case shown="True" w158 {
          tunnel: "Parameter 11" -> [_ w369]
          tunnel: ["" ("format string") w368] -> w156
          tunnel: ["" w367] -> w155
          tunnel: ["" ("date/time string") w366] -> w154
          frame False {
            w353 = u16 0 items=["Choose parameter", "Date", "Time", "Catalog ID"] ("Parameter 11")
            w357 = u16 0 items=["All", "P=V1", "P#V1", "P<V1", "P<=V1", "P>V1", "P>=V1", "V1<P<V2", "V1<=P<V2", "V1<P<=V2", "V1<=P<=V2"] ("Operator 11")
            n334 = property on="Date 12" class="AbsTime (strict)"("Visible"=FALSE) -> ()  [unwired: 2 in, 2 out]
            n335 = property on="Date 11" class="AbsTime (strict)"("Visible"=FALSE) -> ()  [unwired: 2 in, 2 out]
            n336 = property on="Operator 11" class="Ring (strict)"("Value"=w357) -> ()  [unwired: 2 in, 2 out]
            n337 = property on="Parameter 11" class="Ring (strict)"("Value"=w353) -> ()  [unwired: 2 in, 2 out]
            n338 = property on="Catalog ID 12" class="DigNum (strict)"("Visible"=FALSE) -> ()  [unwired: 2 in, 2 out]
            n339 = property on="Catalog ID 11" class="DigNum (strict)"("Visible"=FALSE) -> ()  [unwired: 2 in, 2 out]
            n340 = property on="Value String 11" class="Str"("Visible"=FALSE) -> ()  [unwired: 2 in, 2 out]
            n341 = property on="Value String 12" class="Str"("Visible"=FALSE) -> ()  [unwired: 2 in, 2 out]
            n342 = property on="Time 11" class="AbsTime (strict)"("Visible"=FALSE) -> ()  [unwired: 2 in, 2 out]
            n343 = property on="Time 12" class="AbsTime (strict)"("Visible"=FALSE) -> ()  [unwired: 2 in, 2 out]
          }
          frame True {
            n344 = case shown="3" w369 {
              tunnel: ["" "date" ("format string") "time" ("format string") "catalog_id" ("format string")] -> w368
              tunnel: ["" w386 w409 w428] -> w367
              tunnel: ["" ("date/time string") w385 w407 "" ("date/time string")] -> w366
              frame 0, Default {
                w370 = u16 0 items=["All", "P=V1", "P#V1", "P<V1", "P<=V1", "P>V1", "P>=V1", "V1<P<V2", "V1<=P<V2", "V1<P<=V2", "V1<=P<=V2"] ("Operator 11")
                n345 = property on="Date 12" class="AbsTime (strict)"("Visible"=FALSE) -> ()  [unwired: 2 in, 2 out]
                n346 = property on="Date 11" class="AbsTime (strict)"("Visible"=FALSE) -> ()  [unwired: 2 in, 2 out]
                n347 = property on="Catalog ID 12" class="DigNum (strict)"("Visible"=FALSE) -> ()  [unwired: 2 in, 2 out]
                n348 = property on="Catalog ID 11" class="DigNum (strict)"("Visible"=FALSE) -> ()  [unwired: 2 in, 2 out]
                n349 = property on="Operator 11" class="Ring (strict)"("Disabled Items []"=i32[] [1, 2, 3, 4, 5, 6, 7, 8, 9, 10], "Value"=w370) -> ()  [unwired: 2 in, 2 out]
                n350 = property on="Value String 11" class="Str"("Visible"=TRUE) -> ()  [unwired: 2 in, 2 out]
                n351 = property on="Value String 12" class="Str"("Visible"=TRUE) -> ()  [unwired: 2 in, 2 out]
                n352 = property on="Time 11" class="AbsTime (strict)"("Visible"=FALSE) -> ()  [unwired: 2 in, 2 out]
                n353 = property on="Time 12" class="AbsTime (strict)"("Visible"=FALSE) -> ()  [unwired: 2 in, 2 out]
              }
              frame 1 {
                n354 = property on="Date 12" class="AbsTime (strict)"("Visible"=TRUE) -> ()  [unwired: 2 in, 2 out]
                n355 = property on="Date 11" class="AbsTime (strict)"("Visible"=TRUE) -> ()  [unwired: 2 in, 2 out]
                n356 = property on="Operator 11" class="Ring (strict)"("Disabled Items []"=i32[] []) -> ()  [unwired: 2 in, 2 out]
                n357 = property on="Catalog ID 12" class="DigNum (strict)"("Visible"=FALSE) -> ()  [unwired: 2 in, 2 out]
                n358 = property on="Catalog ID 11" class="DigNum (strict)"("Visible"=FALSE) -> ()  [unwired: 2 in, 2 out]
                n359 = property on="Time 11" class="AbsTime (strict)"("Visible"=FALSE) -> ()  [unwired: 2 in, 2 out]
                n360 = property on="Time 12" class="AbsTime (strict)"("Visible"=FALSE) -> ()  [unwired: 2 in, 2 out]
                n361 = property on="Value String 11" class="Str"("Visible"=FALSE) -> ()  [unwired: 2 in, 2 out]
                n362 = property on="Value String 12" class="Str"("Visible"=FALSE) -> ()  [unwired: 2 in, 2 out]
                n363 = Format Date/Time String(time format string (%c)="%Y/%m/%d", seconds (now)="Date 12") -> (date/time string=w395:string)  [unwired: 1 in]
                n364 = Format Date/Time String(time format string (%c)="%Y/%m/%d", seconds (now)="Date 11") -> (date/time string=w394:string)  [unwired: 1 in]
                n365 = Concatenate Strings("'" ("string"), w394, "'" ("string")) -> (w386:string)
                n366 = Concatenate Strings("'" ("string"), w395, "'" ("string")) -> (w385:string)
              }
              frame 2 {
                n367 = property on="Date 12" class="AbsTime (strict)"("Visible"=FALSE) -> ()  [unwired: 2 in, 2 out]
                n368 = property on="Date 11" class="AbsTime (strict)"("Visible"=FALSE) -> ()  [unwired: 2 in, 2 out]
                n369 = property on="Operator 11" class="Ring (strict)"("Disabled Items []"=i32[] []) -> ()  [unwired: 2 in, 2 out]
                n370 = property on="Catalog ID 12" class="DigNum (strict)"("Visible"=FALSE) -> ()  [unwired: 2 in, 2 out]
                n371 = property on="Catalog ID 11" class="DigNum (strict)"("Visible"=FALSE) -> ()  [unwired: 2 in, 2 out]
                n372 = property on="Value String 11" class="Str"("Visible"=FALSE) -> ()  [unwired: 2 in, 2 out]
                n373 = property on="Value String 12" class="Str"("Visible"=FALSE) -> ()  [unwired: 2 in, 2 out]
                n374 = Format Date/Time String(time format string (%c)="%H:%M:%S", seconds (now)="Time 11") -> (date/time string=w417:string)  [unwired: 1 in]
                n375 = Format Date/Time String(time format string (%c)="%H:%M:%S", seconds (now)="Time 12") -> (date/time string=w416:string)  [unwired: 1 in]
                n376 = property on="Time 11" class="AbsTime (strict)"("Visible"=TRUE) -> ()  [unwired: 2 in, 2 out]
                n377 = property on="Time 12" class="AbsTime (strict)"("Visible"=TRUE) -> ()  [unwired: 2 in, 2 out]
                n378 = Concatenate Strings("'" ("string"), w417, "'" ("string")) -> (w409:string)
                n379 = Concatenate Strings("'" ("string"), w416, "'" ("string")) -> (w407:string)
              }
              frame 3 {
                n380 = property on="Date 12" class="AbsTime (strict)"("Visible"=FALSE) -> ()  [unwired: 2 in, 2 out]
                n381 = property on="Date 11" class="AbsTime (strict)"("Visible"=FALSE) -> ()  [unwired: 2 in, 2 out]
                n382 = property on="Operator 11" class="Ring (strict)"("Disabled Items []"=i32[] [2, 3, 4, 5, 6, 7, 8, 9, 10]) -> ()  [unwired: 2 in, 2 out]
                n383 = property on="Catalog ID 12" class="DigNum (strict)"("Visible"=TRUE) -> ()  [unwired: 2 in, 2 out]
                n384 = property on="Catalog ID 11" class="DigNum (strict)"("Visible"=TRUE) -> ()  [unwired: 2 in, 2 out]
                n385 = property on="Value String 11" class="Str"("Visible"=FALSE) -> ()  [unwired: 2 in, 2 out]
                n386 = property on="Value String 12" class="Str"("Visible"=FALSE) -> ()  [unwired: 2 in, 2 out]
                n387 = property on="Time 11" class="AbsTime (strict)"("Visible"=FALSE) -> ()  [unwired: 2 in, 2 out]
                n388 = property on="Time 12" class="AbsTime (strict)"("Visible"=FALSE) -> ()  [unwired: 2 in, 2 out]
                n389 = Number To Decimal String(number="Catalog ID 11") -> (decimal integer string=w428:string)  [unwired: 1 in]
              }
            }
          }
        }
        n390 = Build Array(w188, w189, w190, w191, w192) -> (w186:bool[])
        n391 = case shown="3" "Parameter 1" {
          tunnel: ["" ("date/time string") w1111 w1123 w1145] -> w182
          tunnel: ["" ("date/time string") w1105 w1124 "" ("date/time string")] -> w181
          tunnel: ["" ("format string") "date" ("format string") "time" ("format string") "catalog_id" ("format string")] -> w180
          frame 0, Default {
            w1088 = u16 0 items=["All", "P=V1", "P#V1", "P<V1", "P<=V1", "P>V1", "P>=V1", "V1<P<V2", "V1<=P<V2", "V1<P<=V2", "V1<=P<=V2"] ("Operator 1")
            n392 = property on="Value String 1" class="Str"("Visible"=TRUE) -> ()  [unwired: 2 in, 2 out]
            n393 = property on="Value String 2" class="Str"("Visible"=TRUE) -> ()  [unwired: 2 in, 2 out]
            n394 = property on="Time 1" class="AbsTime (strict)"("Visible"=FALSE) -> ()  [unwired: 2 in, 2 out]
            n395 = property on="Catalog ID 1" class="DigNum (strict)"("Visible"=FALSE) -> ()  [unwired: 2 in, 2 out]
            n396 = property on="Operator 1" class="Ring (strict)"("Disabled Items []"=i32[] [1, 2, 3, 4, 5, 6, 7, 8, 9, 10], "Value"=w1088) -> ()  [unwired: 2 in, 2 out]
            n397 = property on="Catalog ID 2" class="DigNum (strict)"("Visible"=FALSE) -> ()  [unwired: 2 in, 2 out]
            n398 = property on="Time 2" class="AbsTime (strict)"("Visible"=FALSE) -> ()  [unwired: 2 in, 2 out]
            n399 = property on="Date 1" class="AbsTime (strict)"("Visible"=FALSE) -> ()  [unwired: 2 in, 2 out]
            n400 = property on="Date 2" class="AbsTime (strict)"("Visible"=FALSE) -> ()  [unwired: 2 in, 2 out]
          }
          frame 1 {
            n401 = property on="Date 1" class="AbsTime (strict)"("Visible"=TRUE) -> ()  [unwired: 2 in, 2 out]
            n402 = property on="Date 2" class="AbsTime (strict)"("Visible"=TRUE) -> ()  [unwired: 2 in, 2 out]
            n403 = property on="Operator 1" class="Ring (strict)"("Disabled Items []"=i32[] []) -> ()  [unwired: 2 in, 2 out]
            n404 = property on="Time 1" class="AbsTime (strict)"("Visible"=FALSE) -> ()  [unwired: 2 in, 2 out]
            n405 = property on="Time 2" class="AbsTime (strict)"("Visible"=FALSE) -> ()  [unwired: 2 in, 2 out]
            n406 = property on="Catalog ID 2" class="DigNum (strict)"("Visible"=FALSE) -> ()  [unwired: 2 in, 2 out]
            n407 = property on="Catalog ID 1" class="DigNum (strict)"("Visible"=FALSE) -> ()  [unwired: 2 in, 2 out]
            n408 = Format Date/Time String(time format string (%c)="%Y/%m/%d", seconds (now)="Date 2") -> (date/time string=w1104:string)  [unwired: 1 in]
            n409 = Format Date/Time String(time format string (%c)="%Y/%m/%d", seconds (now)="Date 1") -> (date/time string=w1110:string)  [unwired: 1 in]
            n410 = property on="Value String 1" class="Str"("Visible"=FALSE) -> ()  [unwired: 2 in, 2 out]
            n411 = property on="Value String 2" class="Str"("Visible"=FALSE) -> ()  [unwired: 2 in, 2 out]
            n412 = Concatenate Strings("'" ("string"), w1110, "'" ("string")) -> (w1111:string)
            n413 = Concatenate Strings("'" ("string"), w1104, "'" ("string")) -> (w1105:string)
          }
          frame 2 {
            n414 = property on="Date 1" class="AbsTime (strict)"("Visible"=FALSE) -> ()  [unwired: 2 in, 2 out]
            n415 = property on="Date 2" class="AbsTime (strict)"("Visible"=FALSE) -> ()  [unwired: 2 in, 2 out]
            n416 = property on="Operator 1" class="Ring (strict)"("Disabled Items []"=i32[] []) -> ()  [unwired: 2 in, 2 out]
            n417 = property on="Time 1" class="AbsTime (strict)"("Visible"=TRUE) -> ()  [unwired: 2 in, 2 out]
            n418 = property on="Time 2" class="AbsTime (strict)"("Visible"=TRUE) -> ()  [unwired: 2 in, 2 out]
            n419 = property on="Catalog ID 2" class="DigNum (strict)"("Visible"=FALSE) -> ()  [unwired: 2 in, 2 out]
            n420 = property on="Catalog ID 1" class="DigNum (strict)"("Visible"=FALSE) -> ()  [unwired: 2 in, 2 out]
            n421 = Format Date/Time String(time format string (%c)="%H:%M:%S", seconds (now)="Time 1") -> (date/time string=w1126:string)  [unwired: 1 in]
            n422 = Format Date/Time String(time format string (%c)="%H:%M:%S", seconds (now)="Time 2") -> (date/time string=w1125:string)  [unwired: 1 in]
            n423 = property on="Value String 1" class="Str"("Visible"=FALSE) -> ()  [unwired: 2 in, 2 out]
            n424 = property on="Value String 2" class="Str"("Visible"=FALSE) -> ()  [unwired: 2 in, 2 out]
            n425 = Concatenate Strings("'" ("string"), w1126, "'" ("string")) -> (w1123:string)
            n426 = Concatenate Strings("'" ("string"), w1125, "'" ("string")) -> (w1124:string)
          }
          frame 3 {
            n427 = property on="Date 1" class="AbsTime (strict)"("Visible"=FALSE) -> ()  [unwired: 2 in, 2 out]
            n428 = property on="Date 2" class="AbsTime (strict)"("Visible"=FALSE) -> ()  [unwired: 2 in, 2 out]
            n429 = property on="Operator 1" class="Ring (strict)"("Disabled Items []"=i32[] [2, 3, 4, 5, 6, 7, 8, 9, 10]) -> ()  [unwired: 2 in, 2 out]
            n430 = property on="Time 1" class="AbsTime (strict)"("Visible"=FALSE) -> ()  [unwired: 2 in, 2 out]
            n431 = property on="Time 2" class="AbsTime (strict)"("Visible"=FALSE) -> ()  [unwired: 2 in, 2 out]
            n432 = property on="Catalog ID 2" class="DigNum (strict)"("Visible"=TRUE) -> ()  [unwired: 2 in, 2 out]
            n433 = property on="Catalog ID 1" class="DigNum (strict)"("Visible"=TRUE) -> ()  [unwired: 2 in, 2 out]
            n434 = Number To Decimal String(number="Catalog ID 1") -> (decimal integer string=w1145:string)  [unwired: 1 in]
            n435 = property on="Value String 1" class="Str"("Visible"=FALSE) -> ()  [unwired: 2 in, 2 out]
            n436 = property on="Value String 2" class="Str"("Visible"=FALSE) -> ()  [unwired: 2 in, 2 out]
          }
        }
        n437 = Boolean To (0,1)(Boolean=w186) -> (0, 1=w187:i16[])
        n438 = Add Array Elements(numeric array=w187) -> (sum=w185:i16)
        n439 = case shown="0, Default" w185 {
          frame 0, Default {
            n440 = property on="Parameter 1" class="Ring (strict)"("Visible"=TRUE) -> ()  [unwired: 2 in, 2 out]
            n441 = property on="Operator 1" class="Ring (strict)"("Visible"=TRUE) -> ()  [unwired: 2 in, 2 out]
            n442 = property on="Operator 13" class="Ring (strict)"("Visible"=FALSE) -> ()  [unwired: 2 in, 2 out]
            n443 = property on="Operator 14" class="Ring (strict)"("Visible"=FALSE) -> ()  [unwired: 2 in, 2 out]
            n444 = property on="Parameter 3" class="Ring (strict)"("Visible"=FALSE) -> ()  [unwired: 2 in, 2 out]
            n445 = property on="Operator 3" class="Ring (strict)"("Visible"=FALSE) -> ()  [unwired: 2 in, 2 out]
            n446 = property on="Operator 15" class="Ring (strict)"("Visible"=FALSE) -> ()  [unwired: 2 in, 2 out]
            n447 = property on="Parameter 5" class="Ring (strict)"("Visible"=FALSE) -> ()  [unwired: 2 in, 2 out]
            n448 = property on="Operator 5" class="Ring (strict)"("Visible"=FALSE) -> ()  [unwired: 2 in, 2 out]
            n449 = property on="Operator 16" class="Ring (strict)"("Visible"=FALSE) -> ()  [unwired: 2 in, 2 out]
            n450 = property on="Operator 7" class="Ring (strict)"("Visible"=FALSE) -> ()  [unwired: 2 in, 2 out]
            n451 = property on="Parameter 7" class="Ring (strict)"("Visible"=FALSE) -> ()  [unwired: 2 in, 2 out]
            n452 = property on="Operator 17" class="Ring (strict)"("Visible"=FALSE) -> ()  [unwired: 2 in, 2 out]
            n453 = property on="Operator 9" class="Ring (strict)"("Visible"=FALSE) -> ()  [unwired: 2 in, 2 out]
            n454 = property on="Parameter 9" class="Ring (strict)"("Visible"=FALSE) -> ()  [unwired: 2 in, 2 out]
            n455 = property on="Parameter 11" class="Ring (strict)"("Visible"=FALSE) -> ()  [unwired: 2 in, 2 out]
            n456 = property on="Operator 11" class="Ring (strict)"("Visible"=FALSE) -> ()  [unwired: 2 in, 2 out]
          }
          frame 1 {
            n457 = property on="Operator 13" class="Ring (strict)"("Visible"=TRUE) -> ()  [unwired: 2 in, 2 out]
            n458 = property on="Parameter 1" class="Ring (strict)"("Visible"=TRUE) -> ()  [unwired: 2 in, 2 out]
            n459 = property on="Operator 1" class="Ring (strict)"("Visible"=TRUE) -> ()  [unwired: 2 in, 2 out]
            n460 = property on="Operator 14" class="Ring (strict)"("Visible"=FALSE) -> ()  [unwired: 2 in, 2 out]
            n461 = property on="Parameter 3" class="Ring (strict)"("Visible"=TRUE) -> ()  [unwired: 2 in, 2 out]
            n462 = property on="Operator 3" class="Ring (strict)"("Visible"=TRUE) -> ()  [unwired: 2 in, 2 out]
            n463 = property on="Operator 15" class="Ring (strict)"("Visible"=FALSE) -> ()  [unwired: 2 in, 2 out]
            n464 = property on="Parameter 5" class="Ring (strict)"("Visible"=FALSE) -> ()  [unwired: 2 in, 2 out]
            n465 = property on="Operator 5" class="Ring (strict)"("Visible"=FALSE) -> ()  [unwired: 2 in, 2 out]
            n466 = property on="Operator 16" class="Ring (strict)"("Visible"=FALSE) -> ()  [unwired: 2 in, 2 out]
            n467 = property on="Operator 7" class="Ring (strict)"("Visible"=FALSE) -> ()  [unwired: 2 in, 2 out]
            n468 = property on="Parameter 7" class="Ring (strict)"("Visible"=FALSE) -> ()  [unwired: 2 in, 2 out]
            n469 = property on="Operator 17" class="Ring (strict)"("Visible"=FALSE) -> ()  [unwired: 2 in, 2 out]
            n470 = property on="Operator 9" class="Ring (strict)"("Visible"=FALSE) -> ()  [unwired: 2 in, 2 out]
            n471 = property on="Parameter 9" class="Ring (strict)"("Visible"=FALSE) -> ()  [unwired: 2 in, 2 out]
            n472 = property on="Parameter 11" class="Ring (strict)"("Visible"=FALSE) -> ()  [unwired: 2 in, 2 out]
            n473 = property on="Operator 11" class="Ring (strict)"("Visible"=FALSE) -> ()  [unwired: 2 in, 2 out]
          }
          frame 2 {
            n474 = property on="Parameter 1" class="Ring (strict)"("Visible"=TRUE) -> ()  [unwired: 2 in, 2 out]
            n475 = property on="Operator 1" class="Ring (strict)"("Visible"=TRUE) -> ()  [unwired: 2 in, 2 out]
            n476 = property on="Operator 13" class="Ring (strict)"("Visible"=TRUE) -> ()  [unwired: 2 in, 2 out]
            n477 = property on="Parameter 3" class="Ring (strict)"("Visible"=TRUE) -> ()  [unwired: 2 in, 2 out]
            n478 = property on="Operator 3" class="Ring (strict)"("Visible"=TRUE) -> ()  [unwired: 2 in, 2 out]
            n479 = property on="Operator 14" class="Ring (strict)"("Visible"=TRUE) -> ()  [unwired: 2 in, 2 out]
            n480 = property on="Parameter 5" class="Ring (strict)"("Visible"=TRUE) -> ()  [unwired: 2 in, 2 out]
            n481 = property on="Operator 5" class="Ring (strict)"("Visible"=TRUE) -> ()  [unwired: 2 in, 2 out]
            n482 = property on="Operator 15" class="Ring (strict)"("Visible"=FALSE) -> ()  [unwired: 2 in, 2 out]
            n483 = property on="Operator 7" class="Ring (strict)"("Visible"=FALSE) -> ()  [unwired: 2 in, 2 out]
            n484 = property on="Parameter 7" class="Ring (strict)"("Visible"=FALSE) -> ()  [unwired: 2 in, 2 out]
            n485 = property on="Operator 16" class="Ring (strict)"("Visible"=FALSE) -> ()  [unwired: 2 in, 2 out]
            n486 = property on="Operator 9" class="Ring (strict)"("Visible"=FALSE) -> ()  [unwired: 2 in, 2 out]
            n487 = property on="Parameter 9" class="Ring (strict)"("Visible"=FALSE) -> ()  [unwired: 2 in, 2 out]
            n488 = property on="Operator 17" class="Ring (strict)"("Visible"=FALSE) -> ()  [unwired: 2 in, 2 out]
            n489 = property on="Parameter 11" class="Ring (strict)"("Visible"=FALSE) -> ()  [unwired: 2 in, 2 out]
            n490 = property on="Operator 11" class="Ring (strict)"("Visible"=FALSE) -> ()  [unwired: 2 in, 2 out]
          }
          frame 3 {
            n491 = property on="Parameter 1" class="Ring (strict)"("Visible"=TRUE) -> ()  [unwired: 2 in, 2 out]
            n492 = property on="Operator 1" class="Ring (strict)"("Visible"=TRUE) -> ()  [unwired: 2 in, 2 out]
            n493 = property on="Operator 13" class="Ring (strict)"("Visible"=TRUE) -> ()  [unwired: 2 in, 2 out]
            n494 = property on="Parameter 3" class="Ring (strict)"("Visible"=TRUE) -> ()  [unwired: 2 in, 2 out]
            n495 = property on="Operator 3" class="Ring (strict)"("Visible"=TRUE) -> ()  [unwired: 2 in, 2 out]
            n496 = property on="Operator 14" class="Ring (strict)"("Visible"=TRUE) -> ()  [unwired: 2 in, 2 out]
            n497 = property on="Operator 15" class="Ring (strict)"("Visible"=TRUE) -> ()  [unwired: 2 in, 2 out]
            n498 = property on="Parameter 5" class="Ring (strict)"("Visible"=TRUE) -> ()  [unwired: 2 in, 2 out]
            n499 = property on="Operator 5" class="Ring (strict)"("Visible"=TRUE) -> ()  [unwired: 2 in, 2 out]
            n500 = property on="Operator 16" class="Ring (strict)"("Visible"=FALSE) -> ()  [unwired: 2 in, 2 out]
            n501 = property on="Operator 7" class="Ring (strict)"("Visible"=TRUE) -> ()  [unwired: 2 in, 2 out]
            n502 = property on="Parameter 7" class="Ring (strict)"("Visible"=TRUE) -> ()  [unwired: 2 in, 2 out]
            n503 = property on="Operator 9" class="Ring (strict)"("Visible"=FALSE) -> ()  [unwired: 2 in, 2 out]
            n504 = property on="Parameter 9" class="Ring (strict)"("Visible"=FALSE) -> ()  [unwired: 2 in, 2 out]
            n505 = property on="Operator 17" class="Ring (strict)"("Visible"=FALSE) -> ()  [unwired: 2 in, 2 out]
            n506 = property on="Parameter 11" class="Ring (strict)"("Visible"=FALSE) -> ()  [unwired: 2 in, 2 out]
            n507 = property on="Operator 11" class="Ring (strict)"("Visible"=FALSE) -> ()  [unwired: 2 in, 2 out]
          }
          frame 4 {
            n508 = property on="Operator 13" class="Ring (strict)"("Visible"=TRUE) -> ()  [unwired: 2 in, 2 out]
            n509 = property on="Parameter 1" class="Ring (strict)"("Visible"=TRUE) -> ()  [unwired: 2 in, 2 out]
            n510 = property on="Operator 1" class="Ring (strict)"("Visible"=TRUE) -> ()  [unwired: 2 in, 2 out]
            n511 = property on="Operator 14" class="Ring (strict)"("Visible"=TRUE) -> ()  [unwired: 2 in, 2 out]
            n512 = property on="Parameter 3" class="Ring (strict)"("Visible"=TRUE) -> ()  [unwired: 2 in, 2 out]
            n513 = property on="Operator 3" class="Ring (strict)"("Visible"=TRUE) -> ()  [unwired: 2 in, 2 out]
            n514 = property on="Operator 15" class="Ring (strict)"("Visible"=TRUE) -> ()  [unwired: 2 in, 2 out]
            n515 = property on="Parameter 5" class="Ring (strict)"("Visible"=TRUE) -> ()  [unwired: 2 in, 2 out]
            n516 = property on="Operator 5" class="Ring (strict)"("Visible"=TRUE) -> ()  [unwired: 2 in, 2 out]
            n517 = property on="Operator 16" class="Ring (strict)"("Visible"=TRUE) -> ()  [unwired: 2 in, 2 out]
            n518 = property on="Operator 7" class="Ring (strict)"("Visible"=TRUE) -> ()  [unwired: 2 in, 2 out]
            n519 = property on="Parameter 7" class="Ring (strict)"("Visible"=TRUE) -> ()  [unwired: 2 in, 2 out]
            n520 = property on="Operator 17" class="Ring (strict)"("Visible"=FALSE) -> ()  [unwired: 2 in, 2 out]
            n521 = property on="Operator 9" class="Ring (strict)"("Visible"=TRUE) -> ()  [unwired: 2 in, 2 out]
            n522 = property on="Parameter 9" class="Ring (strict)"("Visible"=TRUE) -> ()  [unwired: 2 in, 2 out]
            n523 = property on="Parameter 11" class="Ring (strict)"("Visible"=FALSE) -> ()  [unwired: 2 in, 2 out]
            n524 = property on="Operator 11" class="Ring (strict)"("Visible"=FALSE) -> ()  [unwired: 2 in, 2 out]
          }
          frame 5 {
            n525 = property on="Parameter 1" class="Ring (strict)"("Visible"=TRUE) -> ()  [unwired: 2 in, 2 out]
            n526 = property on="Operator 1" class="Ring (strict)"("Visible"=TRUE) -> ()  [unwired: 2 in, 2 out]
            n527 = property on="Operator 13" class="Ring (strict)"("Visible"=TRUE) -> ()  [unwired: 2 in, 2 out]
            n528 = property on="Operator 14" class="Ring (strict)"("Visible"=TRUE) -> ()  [unwired: 2 in, 2 out]
            n529 = property on="Parameter 3" class="Ring (strict)"("Visible"=TRUE) -> ()  [unwired: 2 in, 2 out]
            n530 = property on="Operator 3" class="Ring (strict)"("Visible"=TRUE) -> ()  [unwired: 2 in, 2 out]
            n531 = property on="Operator 15" class="Ring (strict)"("Visible"=TRUE) -> ()  [unwired: 2 in, 2 out]
            n532 = property on="Parameter 5" class="Ring (strict)"("Visible"=TRUE) -> ()  [unwired: 2 in, 2 out]
            n533 = property on="Operator 5" class="Ring (strict)"("Visible"=TRUE) -> ()  [unwired: 2 in, 2 out]
            n534 = property on="Operator 16" class="Ring (strict)"("Visible"=TRUE) -> ()  [unwired: 2 in, 2 out]
            n535 = property on="Operator 7" class="Ring (strict)"("Visible"=TRUE) -> ()  [unwired: 2 in, 2 out]
            n536 = property on="Parameter 7" class="Ring (strict)"("Visible"=TRUE) -> ()  [unwired: 2 in, 2 out]
            n537 = property on="Operator 17" class="Ring (strict)"("Visible"=TRUE) -> ()  [unwired: 2 in, 2 out]
            n538 = property on="Operator 9" class="Ring (strict)"("Visible"=TRUE) -> ()  [unwired: 2 in, 2 out]
            n539 = property on="Parameter 9" class="Ring (strict)"("Visible"=TRUE) -> ()  [unwired: 2 in, 2 out]
            n540 = property on="Parameter 11" class="Ring (strict)"("Visible"=TRUE) -> ()  [unwired: 2 in, 2 out]
            n541 = property on="Operator 11" class="Ring (strict)"("Visible"=TRUE) -> ()  [unwired: 2 in, 2 out]
          }
        }
        n542 = case shown="0..6, Default" "Operator 1" {
          frame 0..6, Default {
            w1086 = T1."Disabled and Grayed Out" ("Disabled")
            n543 = property on="Catalog ID 2" class="DigNum (strict)"("DisabledEnum"=w1086) -> ()  [unwired: 2 in, 2 out]
            n544 = property on="Value String 2" class="Str"("DisabledEnum"=w1086) -> ()  [unwired: 2 in, 2 out]
            n545 = property on="Time 2" class="AbsTime (strict)"("DisabledEnum"=w1086) -> ()  [unwired: 2 in, 2 out]
            n546 = property on="Date 2" class="AbsTime (strict)"("DisabledEnum"=w1086) -> ()  [unwired: 2 in, 2 out]
          }
          frame 7..10 {
            w1087 = T1."Enabled" ("Disabled")
            n547 = property on="Catalog ID 2" class="DigNum (strict)"("DisabledEnum"=w1087) -> ()  [unwired: 2 in, 2 out]
            n548 = property on="Value String 2" class="Str"("DisabledEnum"=w1087) -> ()  [unwired: 2 in, 2 out]
            n549 = property on="Time 2" class="AbsTime (strict)"("DisabledEnum"=w1087) -> ()  [unwired: 2 in, 2 out]
            n550 = property on="Date 2" class="AbsTime (strict)"("DisabledEnum"=w1087) -> ()  [unwired: 2 in, 2 out]
          }
        }
        n551 = case shown="7..10" "Operator 3" {
          frame 0..6, Default {
            w924 = T1."Disabled and Grayed Out" ("Disabled")
            n552 = property on="Catalog ID 4" class="DigNum (strict)"("DisabledEnum"=w924) -> ()  [unwired: 2 in, 2 out]
            n553 = property on="Value String 4" class="Str"("DisabledEnum"=w924) -> ()  [unwired: 2 in, 2 out]
            n554 = property on="Time 4" class="AbsTime (strict)"("DisabledEnum"=w924) -> ()  [unwired: 2 in, 2 out]
            n555 = property on="Date 4" class="AbsTime (strict)"("DisabledEnum"=w924) -> ()  [unwired: 2 in, 2 out]
          }
          frame 7..10 {
            w925 = T1."Enabled" ("Disabled")
            n556 = property on="Catalog ID 4" class="DigNum (strict)"("DisabledEnum"=w925) -> ()  [unwired: 2 in, 2 out]
            n557 = property on="Value String 4" class="Str"("DisabledEnum"=w925) -> ()  [unwired: 2 in, 2 out]
            n558 = property on="Time 4" class="AbsTime (strict)"("DisabledEnum"=w925) -> ()  [unwired: 2 in, 2 out]
            n559 = property on="Date 4" class="AbsTime (strict)"("DisabledEnum"=w925) -> ()  [unwired: 2 in, 2 out]
          }
        }
        n560 = case shown="0..6, Default" "Operator 7" {
          frame 0..6, Default {
            w527 = T1."Disabled and Grayed Out" ("Disabled")
            n561 = property on="Catalog ID 8" class="DigNum (strict)"("DisabledEnum"=w527) -> ()  [unwired: 2 in, 2 out]
            n562 = property on="Value String 8" class="Str"("DisabledEnum"=w527) -> ()  [unwired: 2 in, 2 out]
            n563 = property on="Time 8" class="AbsTime (strict)"("DisabledEnum"=w527) -> ()  [unwired: 2 in, 2 out]
            n564 = property on="Date 8" class="AbsTime (strict)"("DisabledEnum"=w527) -> ()  [unwired: 2 in, 2 out]
          }
          frame 7..10 {
            w528 = T1."Enabled" ("Disabled")
            n565 = property on="Catalog ID 8" class="DigNum (strict)"("DisabledEnum"=w528) -> ()  [unwired: 2 in, 2 out]
            n566 = property on="Value String 8" class="Str"("DisabledEnum"=w528) -> ()  [unwired: 2 in, 2 out]
            n567 = property on="Time 8" class="AbsTime (strict)"("DisabledEnum"=w528) -> ()  [unwired: 2 in, 2 out]
            n568 = property on="Date 8" class="AbsTime (strict)"("DisabledEnum"=w528) -> ()  [unwired: 2 in, 2 out]
          }
        }
        n569 = case shown="7..10" "Operator 5" {
          frame 0..6, Default {
            w835 = T1."Disabled and Grayed Out" ("Disabled")
            n570 = property on="Catalog ID 6" class="DigNum (strict)"("DisabledEnum"=w835) -> ()  [unwired: 2 in, 2 out]
            n571 = property on="Value String 6" class="Str"("DisabledEnum"=w835) -> ()  [unwired: 2 in, 2 out]
            n572 = property on="Time 6" class="AbsTime (strict)"("DisabledEnum"=w835) -> ()  [unwired: 2 in, 2 out]
            n573 = property on="Date 6" class="AbsTime (strict)"("DisabledEnum"=w835) -> ()  [unwired: 2 in, 2 out]
          }
          frame 7..10 {
            w836 = T1."Enabled" ("Disabled")
            n574 = property on="Catalog ID 6" class="DigNum (strict)"("DisabledEnum"=w836) -> ()  [unwired: 2 in, 2 out]
            n575 = property on="Value String 6" class="Str"("DisabledEnum"=w836) -> ()  [unwired: 2 in, 2 out]
            n576 = property on="Time 6" class="AbsTime (strict)"("DisabledEnum"=w836) -> ()  [unwired: 2 in, 2 out]
            n577 = property on="Date 6" class="AbsTime (strict)"("DisabledEnum"=w836) -> ()  [unwired: 2 in, 2 out]
          }
        }
        n578 = case shown="1" "Operator 1" {
          tunnel: w182 -> [_ w1017 w1023 w1029 w1035 w1041 w1047 w1057 w1063 w1072 w1081]
          tunnel: w181 -> [_ _ _ _ _ _ _ w1053 w1062 w1071 w1080]
          tunnel: w180 -> [_ w1019 w1024 w1030 w1036 w1042 w1048 w1055 w1064 w1073 w1082]
          tunnel: ["( TRUE )" w1016 w1022 w1028 w1034 w1040 w1046 w1052 w1061 w1070 w1079] -> w145
          frame 0, Default {
          }
          frame 1 {
            n579 = Concatenate Strings("( " ("string"), w1019, " = " ("string"), w1017, " )" ("string")) -> (w1016:string)
          }
          frame 2 {
            n580 = Concatenate Strings("( " ("string"), w1024, " != " ("string"), w1023, " )" ("string")) -> (w1022:string)
          }
          frame 3 {
            n581 = Concatenate Strings("( " ("string"), w1030, " < " ("string"), w1029, " )" ("string")) -> (w1028:string)
          }
          frame 4 {
            n582 = Concatenate Strings("( " ("string"), w1036, " <= " ("string"), w1035, " )" ("string")) -> (w1034:string)
          }
          frame 5 {
            n583 = Concatenate Strings("( " ("string"), w1042, " > " ("string"), w1041, " )" ("string")) -> (w1040:string)
          }
          frame 6 {
            n584 = Concatenate Strings("( " ("string"), w1048, " >= " ("string"), w1047, " )" ("string")) -> (w1046:string)
          }
          frame 7 {
            n585 = Concatenate Strings("( " ("string"), w1055, " > " ("string"), w1057, " AND " ("string"), w1055, " < " ("string"), w1053, " )" ("string")) -> (w1052:string)
          }
          frame 8 {
            n586 = Concatenate Strings("( " ("string"), w1064, " >= " ("string"), w1063, " AND " ("string"), w1064, " < " ("string"), w1062, " )" ("string")) -> (w1061:string)
          }
          frame 9 {
            n587 = Concatenate Strings("( " ("string"), w1073, " > " ("string"), w1072, " AND " ("string"), w1073, " <= " ("string"), w1071, " )" ("string")) -> (w1070:string)
          }
          frame 10 {
            n588 = Concatenate Strings("( " ("string"), w1082, " >= " ("string"), w1081, " AND " ("string"), w1082, " <= " ("string"), w1080, " )" ("string")) -> (w1079:string)
          }
        }
        n589 = case shown="0, Default" "Operator 3" {
          tunnel: w170 -> [_ w766 w772 w778 w784 w790 w796 w806 w812 w821 w830]
          tunnel: w169 -> [_ _ _ _ _ _ _ w802 w811 w820 w829]
          tunnel: w171 -> [_ w768 w773 w779 w785 w791 w797 w804 w813 w822 w831]
          tunnel: ["( TRUE )" w765 w771 w777 w783 w789 w795 w801 w810 w819 w828] -> w143
          frame 0, Default {
          }
          frame 1 {
            n590 = Concatenate Strings("( " ("string"), w768, " = " ("string"), w766, " )" ("string")) -> (w765:string)
          }
          frame 2 {
            n591 = Concatenate Strings("( " ("string"), w773, " != " ("string"), w772, " )" ("string")) -> (w771:string)
          }
          frame 3 {
            n592 = Concatenate Strings("( " ("string"), w779, " < " ("string"), w778, " )" ("string")) -> (w777:string)
          }
          frame 4 {
            n593 = Concatenate Strings("( " ("string"), w785, " <= " ("string"), w784, " )" ("string")) -> (w783:string)
          }
          frame 5 {
            n594 = Concatenate Strings("( " ("string"), w791, " > " ("string"), w790, " )" ("string")) -> (w789:string)
          }
          frame 6 {
            n595 = Concatenate Strings("( " ("string"), w797, " >= " ("string"), w796, " )" ("string")) -> (w795:string)
          }
          frame 7 {
            n596 = Concatenate Strings("( " ("string"), w804, " > " ("string"), w806, " AND " ("string"), w804, " < " ("string"), w802, " )" ("string")) -> (w801:string)
          }
          frame 8 {
            n597 = Concatenate Strings("( " ("string"), w813, " >= " ("string"), w812, " AND " ("string"), w813, " < " ("string"), w811, " )" ("string")) -> (w810:string)
          }
          frame 9 {
            n598 = Concatenate Strings("( " ("string"), w822, " > " ("string"), w821, " AND " ("string"), w822, " <= " ("string"), w820, " )" ("string")) -> (w819:string)
          }
          frame 10 {
            n599 = Concatenate Strings("( " ("string"), w831, " >= " ("string"), w830, " AND " ("string"), w831, " <= " ("string"), w829, " )" ("string")) -> (w828:string)
          }
        }
        n600 = case shown="0, Default" "Operator 7" {
          tunnel: w161 -> [_ w533 w539 w545 w551 w557 w563 w573 w579 w588 w597]
          tunnel: w160 -> [_ _ _ _ _ _ _ w569 w578 w587 w596]
          tunnel: w162 -> [_ w535 w540 w546 w552 w558 w564 w571 w580 w589 w598]
          tunnel: ["( TRUE )" w532 w538 w544 w550 w556 w562 w568 w577 w586 w595] -> w129
          frame 0, Default {
          }
          frame 1 {
            n601 = Concatenate Strings("( " ("string"), w535, " = " ("string"), w533, " )" ("string")) -> (w532:string)
          }
          frame 2 {
            n602 = Concatenate Strings("( " ("string"), w540, " != " ("string"), w539, " )" ("string")) -> (w538:string)
          }
          frame 3 {
            n603 = Concatenate Strings("( " ("string"), w546, " < " ("string"), w545, " )" ("string")) -> (w544:string)
          }
          frame 4 {
            n604 = Concatenate Strings("( " ("string"), w552, " <= " ("string"), w551, " )" ("string")) -> (w550:string)
          }
          frame 5 {
            n605 = Concatenate Strings("( " ("string"), w558, " > " ("string"), w557, " )" ("string")) -> (w556:string)
          }
          frame 6 {
            n606 = Concatenate Strings("( " ("string"), w564, " >= " ("string"), w563, " )" ("string")) -> (w562:string)
          }
          frame 7 {
            n607 = Concatenate Strings("( " ("string"), w571, " > " ("string"), w573, " AND " ("string"), w571, " < " ("string"), w569, " )" ("string")) -> (w568:string)
          }
          frame 8 {
            n608 = Concatenate Strings("( " ("string"), w580, " >= " ("string"), w579, " AND " ("string"), w580, " < " ("string"), w578, " )" ("string")) -> (w577:string)
          }
          frame 9 {
            n609 = Concatenate Strings("( " ("string"), w589, " > " ("string"), w588, " AND " ("string"), w589, " <= " ("string"), w587, " )" ("string")) -> (w586:string)
          }
          frame 10 {
            n610 = Concatenate Strings("( " ("string"), w598, " >= " ("string"), w597, " AND " ("string"), w598, " <= " ("string"), w596, " )" ("string")) -> (w595:string)
          }
        }
        n611 = case shown="0, Default" "Operator 5" {
          tunnel: w166 -> [_ w693 w699 w705 w711 w717 w723 w733 w739 w748 w757]
          tunnel: w165 -> [_ _ _ _ _ _ _ w729 w738 w747 w756]
          tunnel: w167 -> [_ w695 w700 w706 w712 w718 w724 w731 w740 w749 w758]
          tunnel: ["( TRUE )" w692 w698 w704 w710 w716 w722 w728 w737 w746 w755] -> w127
          frame 0, Default {
          }
          frame 1 {
            n612 = Concatenate Strings("( " ("string"), w695, " = " ("string"), w693, " )" ("string")) -> (w692:string)
          }
          frame 2 {
            n613 = Concatenate Strings("( " ("string"), w700, " != " ("string"), w699, " )" ("string")) -> (w698:string)
          }
          frame 3 {
            n614 = Concatenate Strings("( " ("string"), w706, " < " ("string"), w705, " )" ("string")) -> (w704:string)
          }
          frame 4 {
            n615 = Concatenate Strings("( " ("string"), w712, " <= " ("string"), w711, " )" ("string")) -> (w710:string)
          }
          frame 5 {
            n616 = Concatenate Strings("( " ("string"), w718, " > " ("string"), w717, " )" ("string")) -> (w716:string)
          }
          frame 6 {
            n617 = Concatenate Strings("( " ("string"), w724, " >= " ("string"), w723, " )" ("string")) -> (w722:string)
          }
          frame 7 {
            n618 = Concatenate Strings("( " ("string"), w731, " > " ("string"), w733, " AND " ("string"), w731, " < " ("string"), w729, " )" ("string")) -> (w728:string)
          }
          frame 8 {
            n619 = Concatenate Strings("( " ("string"), w740, " >= " ("string"), w739, " AND " ("string"), w740, " < " ("string"), w738, " )" ("string")) -> (w737:string)
          }
          frame 9 {
            n620 = Concatenate Strings("( " ("string"), w749, " > " ("string"), w748, " AND " ("string"), w749, " <= " ("string"), w747, " )" ("string")) -> (w746:string)
          }
          frame 10 {
            n621 = Concatenate Strings("( " ("string"), w758, " >= " ("string"), w757, " AND " ("string"), w758, " <= " ("string"), w756, " )" ("string")) -> (w755:string)
          }
        }
        n622 = case shown="7..10" "Operator 9" {
          frame 0..6, Default {
            w203 = T1."Disabled and Grayed Out" ("Disabled")
            n623 = property on="Catalog ID 10" class="DigNum (strict)"("DisabledEnum"=w203) -> ()  [unwired: 2 in, 2 out]
            n624 = property on="Value String 10" class="Str"("DisabledEnum"=w203) -> ()  [unwired: 2 in, 2 out]
            n625 = property on="Time 10" class="AbsTime (strict)"("DisabledEnum"=w203) -> ()  [unwired: 2 in, 2 out]
            n626 = property on="Date 10" class="AbsTime (strict)"("DisabledEnum"=w203) -> ()  [unwired: 2 in, 2 out]
          }
          frame 7..10 {
            w204 = T1."Enabled" ("Disabled")
            n627 = property on="Catalog ID 10" class="DigNum (strict)"("DisabledEnum"=w204) -> ()  [unwired: 2 in, 2 out]
            n628 = property on="Value String 10" class="Str"("DisabledEnum"=w204) -> ()  [unwired: 2 in, 2 out]
            n629 = property on="Time 10" class="AbsTime (strict)"("DisabledEnum"=w204) -> ()  [unwired: 2 in, 2 out]
            n630 = property on="Date 10" class="AbsTime (strict)"("DisabledEnum"=w204) -> ()  [unwired: 2 in, 2 out]
          }
        }
        n631 = case shown="7..10" "Operator 11" {
          frame 0..6, Default {
            w351 = T1."Disabled and Grayed Out" ("Disabled")
            n632 = property on="Catalog ID 12" class="DigNum (strict)"("DisabledEnum"=w351) -> ()  [unwired: 2 in, 2 out]
            n633 = property on="Value String 12" class="Str"("DisabledEnum"=w351) -> ()  [unwired: 2 in, 2 out]
            n634 = property on="Time 12" class="AbsTime (strict)"("DisabledEnum"=w351) -> ()  [unwired: 2 in, 2 out]
            n635 = property on="Date 12" class="AbsTime (strict)"("DisabledEnum"=w351) -> ()  [unwired: 2 in, 2 out]
          }
          frame 7..10 {
            w352 = T1."Enabled" ("Disabled")
            n636 = property on="Catalog ID 12" class="DigNum (strict)"("DisabledEnum"=w352) -> ()  [unwired: 2 in, 2 out]
            n637 = property on="Value String 12" class="Str"("DisabledEnum"=w352) -> ()  [unwired: 2 in, 2 out]
            n638 = property on="Time 12" class="AbsTime (strict)"("DisabledEnum"=w352) -> ()  [unwired: 2 in, 2 out]
            n639 = property on="Date 12" class="AbsTime (strict)"("DisabledEnum"=w352) -> ()  [unwired: 2 in, 2 out]
          }
        }
        n640 = case shown="0, Default" "Operator 9" {
          tunnel: w151 -> [_ w209 w215 w221 w227 w233 w239 w249 w255 w264 w273]
          tunnel: w150 -> [_ _ _ _ _ _ _ w245 w254 w263 w272]
          tunnel: w152 -> [_ w211 w216 w222 w228 w234 w240 w247 w256 w265 w274]
          tunnel: ["( TRUE )" w208 w214 w220 w226 w232 w238 w244 w253 w262 w271] -> w124
          frame 0, Default {
          }
          frame 1 {
            n641 = Concatenate Strings("( " ("string"), w211, " = " ("string"), w209, " )" ("string")) -> (w208:string)
          }
          frame 2 {
            n642 = Concatenate Strings("( " ("string"), w216, " != " ("string"), w215, " )" ("string")) -> (w214:string)
          }
          frame 3 {
            n643 = Concatenate Strings("( " ("string"), w222, " < " ("string"), w221, " )" ("string")) -> (w220:string)
          }
          frame 4 {
            n644 = Concatenate Strings("( " ("string"), w228, " <= " ("string"), w227, " )" ("string")) -> (w226:string)
          }
          frame 5 {
            n645 = Concatenate Strings("( " ("string"), w234, " > " ("string"), w233, " )" ("string")) -> (w232:string)
          }
          frame 6 {
            n646 = Concatenate Strings("( " ("string"), w240, " >= " ("string"), w239, " )" ("string")) -> (w238:string)
          }
          frame 7 {
            n647 = Concatenate Strings("( " ("string"), w247, " > " ("string"), w249, " AND " ("string"), w247, " < " ("string"), w245, " )" ("string")) -> (w244:string)
          }
          frame 8 {
            n648 = Concatenate Strings("( " ("string"), w256, " >= " ("string"), w255, " AND " ("string"), w256, " < " ("string"), w254, " )" ("string")) -> (w253:string)
          }
          frame 9 {
            n649 = Concatenate Strings("( " ("string"), w265, " > " ("string"), w264, " AND " ("string"), w265, " <= " ("string"), w263, " )" ("string")) -> (w262:string)
          }
          frame 10 {
            n650 = Concatenate Strings("( " ("string"), w274, " >= " ("string"), w273, " AND " ("string"), w274, " <= " ("string"), w272, " )" ("string")) -> (w271:string)
          }
        }
        n651 = case shown="0, Default" "Operator 11" {
          tunnel: w155 -> [_ w282 w288 w294 w300 w306 w312 w322 w328 w337 w346]
          tunnel: w154 -> [_ _ _ _ _ _ _ w318 w327 w336 w345]
          tunnel: w156 -> [_ w284 w289 w295 w301 w307 w313 w320 w329 w338 w347]
          tunnel: ["( TRUE )" w281 w287 w293 w299 w305 w311 w317 w326 w335 w344] -> w119
          frame 0, Default {
          }
          frame 1 {
            n652 = Concatenate Strings("( " ("string"), w284, " = " ("string"), w282, " )" ("string")) -> (w281:string)
          }
          frame 2 {
            n653 = Concatenate Strings("( " ("string"), w289, " != " ("string"), w288, " )" ("string")) -> (w287:string)
          }
          frame 3 {
            n654 = Concatenate Strings("( " ("string"), w295, " < " ("string"), w294, " )" ("string")) -> (w293:string)
          }
          frame 4 {
            n655 = Concatenate Strings("( " ("string"), w301, " <= " ("string"), w300, " )" ("string")) -> (w299:string)
          }
          frame 5 {
            n656 = Concatenate Strings("( " ("string"), w307, " > " ("string"), w306, " )" ("string")) -> (w305:string)
          }
          frame 6 {
            n657 = Concatenate Strings("( " ("string"), w313, " >= " ("string"), w312, " )" ("string")) -> (w311:string)
          }
          frame 7 {
            n658 = Concatenate Strings("( " ("string"), w320, " > " ("string"), w322, " AND " ("string"), w320, " < " ("string"), w318, " )" ("string")) -> (w317:string)
          }
          frame 8 {
            n659 = Concatenate Strings("( " ("string"), w329, " >= " ("string"), w328, " AND " ("string"), w329, " < " ("string"), w327, " )" ("string")) -> (w326:string)
          }
          frame 9 {
            n660 = Concatenate Strings("( " ("string"), w338, " > " ("string"), w337, " AND " ("string"), w338, " <= " ("string"), w336, " )" ("string")) -> (w335:string)
          }
          frame 10 {
            n661 = Concatenate Strings("( " ("string"), w347, " >= " ("string"), w346, " AND " ("string"), w347, " <= " ("string"), w345, " )" ("string")) -> (w344:string)
          }
        }
        n662 = case shown="0, Default" "Operator 13" {
          tunnel: [" AND " " OR "] -> w148
          frame 0, Default {
          }
          frame 1 {
          }
        }
        n663 = case shown="0, Default" "Operator 15" {
          tunnel: [" AND " " OR "] -> w135
          frame 0, Default {
          }
          frame 1 {
          }
        }
        n664 = case shown="0, Default" "Operator 14" {
          tunnel: [" AND " " OR "] -> w141
          frame 0, Default {
          }
          frame 1 {
          }
        }
        n665 = property on="sub 1" class="Bool"() -> ("Visible"=w146:bool)  [unwired: 2 in, 2 out]
        n666 = property on="sub 3" class="Bool"() -> ("Visible"=w134:bool)  [unwired: 2 in, 2 out]
        n667 = property on="sub 2" class="Bool"() -> ("Visible"=w139:bool)  [unwired: 2 in, 2 out]
        n668 = case shown="0, Default" "Operator 16" {
          tunnel: [" AND " " OR "] -> w130
          frame 0, Default {
          }
          frame 1 {
          }
        }
        n669 = property on="sub 4" class="Bool"() -> ("Visible"=w132:bool)  [unwired: 2 in, 2 out]
        n670 = property on="sub 5" class="Bool"() -> ("Visible"=w122:bool)  [unwired: 2 in, 2 out]
        n671 = case shown="0, Default" "Operator 17" {
          tunnel: [" AND " " OR "] -> w121
          frame 0, Default {
          }
          frame 1 {
          }
        }
        n672 = Select(t=w141, s=w139, f=" AND ") -> (s? t:f=w138:string)
        n673 = Select(t=w148, s=w146, f=" AND ") -> (s? t:f=w144:string)
        n674 = Select(t=w135, s=w134, f=" AND ") -> (s? t:f=w126:string)
        n675 = Select(t=w130, s=w132, f=" AND ") -> (s? t:f=w125:string)
        n676 = Select(t=w121, s=w122, f=" AND ") -> (s? t:f=w120:string)
        n677 = Concatenate Strings("WHERE " ("string"), w145, w144, w143, w138, w127, w126, w129, w125, w124, w120, w119, " ORDER BY id DESC" ("string")) -> (→"Query String":string)
      }
    }
  }
  n678 = shared-variable ".\\database.lvlib\\search"(FALSE ("search")) -> ()  [unwired: 1 in, 1 out]
  "String 1" <- "Value 1" ("String 1")
  "String 2" <- "Value 2" ("String 2")
  "String 3" <- "Operation" ("String 1")
  "String 4" <- "Parameter" ("String 4")
  "Value String 1" <- "Value" ("Value String 1")
  "Value String 2" <- "Value" ("Value String 2")
  "Value String 3" <- "Value" ("Value String 3")
  "Value String 4" <- "Value" ("Value String 4")
  "Value String 5" <- "Value" ("Value String 5")
  "Value String 6" <- "Value" ("Value String 6")
  "Value String 7" <- "Value" ("Value String 7")
  "Value String 8" <- "Value" ("Value String 8")
  "Value String 9" <- "Value" ("Value String 9")
  "Value String 10" <- "Value" ("Value String 10")
  "Value String 11" <- "Value" ("Value String 11")
  "Value String 12" <- "Value" ("Value String 12")
  "Name" <- "Search in Database" ("Name")
